vi "Tool-BLED112 GUI IntervalTime Cal.vi"() -> ()   [LabVIEW 2015]
uses:
  <vilib>/Analysis/baseanly.llb/Mean (DBL).vi
  <vilib>/Analysis/NI_AALBase.lvlib
panel:
  out "전체 시간(s)":dbl=17.30500000000029 format="%0.2f"
  out "평균 Interval time(ms)":dbl=49.87031700288185 format="%0.2f"
  out "Packet Length":i32=349
  out "Interval time":dbl(graph)=3.0
  in  "Log data &bled gui":string="2016.08.18 17:13:00.655 ble_evt_attclient_attribute_value connection: 0 (0x00) atthandle: 11 (0x000b) type: 1 (0x01) value:1fe8952003fc1fd90f20421d205d8a201abb0100\n2016.08.18 17:13:00.657 RX: 80190405000b0001141fe8952003fc1fd90f20421d205d8a201abb0100\n\n2016.08.18 17:13:00.658 ble_evt_attclient_attribute_value connection: 0 (0x00) atthandle: 15 (0x000f) type: 1 (0x01) value:02bcfe33fe4b0158ff4241a70000000000000000\n2016.08.18 17:13:00.659 RX: 80190405000f00011402bcfe33fe4b0158ff4241a70000000000000000\n\n2016.08.18 17:13:00.753 ble_evt_attclient_attribute_value connection: 0 (0x00) atthandle: 11 (0x000b) type: 1 (0x01) value:1fe8952003fa1fd910204218205d87201abe0100\n2016.08.18 17:13:00.754 RX: 80190405000b0001141fe8952003fa1fd910204218205d87201abe0100\n\n2016.08.18 17:13:00.758 ble_evt_attclient_attribute_value connection: 0 (0x00) atthandle: 15 (0x000f) type: 1 (0x01) value:02c4fe29fe48013bff5b41ac0000000000000000\n2016.08.18 17:13:00.759 RX: 80190405000f00011402c4fe29fe48013bff5b41ac0000000000000000\n\n2016.08.18 17:13:00.858 ble_evt_attclient_attribute_value connection: 0 (0x00) atthandle: 11 (0x000b) type: 1 (0x01) value:1fe8932003f91fd90e204217205d83201abc0100\n2016.08.18 17:13:00.859 RX: 80190405000b0001141fe8932003f91fd90e204217205d83201abc0100\n\n2016.08.18 17:13:00.860 ble_evt_attclient_attribute_value connection: 0 (0x00) atthandle: 15 (0x000f) type: 1 (0x01) value:02c8fe2efe470135ff6341b80000000000000000\n2016.08.18 17:13:00.862 RX: 80190405000f00011402c8fe2efe470135ff6341b80000000000000000\n\n2016.08.18 17:13:00.955 ble_evt_attclient_attribute_value connection: 0 (0x00) atthandle: 11 (0x000b) type: 1 (0x01) value:1fe8922003f51fd915204218205d87201aba0100\n2016.08.18 17:13:00.957 RX: 80190405000b0001141fe8922003f51fd915204218205d87201aba0100\n\n2016.08.18 17:13:00.958 ble_evt_attclient_attribute_value connection: 0 (0x00) atthandle: 15 (0x000f) type: 1 (0x01) value:02c8fe27fe4b013dff4741b70000000000000000\n2016.08.18 17:13:00.959 RX: 80190405000f00011402c8fe27fe4b013dff4741b70000000000000000\n\n2016.08.18 17:13:01.053 ble_evt_attclient_attribute_value connection: 0 (0x00) atthandle: 11 (0x000b) type: 1 (0x01) value:1fe8a02003f91fd91820421a205d8b201ab70100\n2016.08.18 17:13:01.055 RX: 80190405000b0001141fe8a02003f91fd91820421a205d8b201ab70100\n\n2016.08.18 17:13:01.060 ble_evt_attclient_attribute_value connection: 0 (0x00) atthandle: 15 (0x000f) type: 1 (0x01) value:02bbfe24fe4c0149ff2641b80000000000000000\n2016.08.18 17:13:01.061 RX: 80190405000f00011402bbfe24fe4c0149ff2641b80000000000000000\n\n2016.08.18 17:13:01.158 ble_evt_attclient_attribute_value connection: 0 (0x00) atthandle: 11 (0x000b) type: 1 (0x01) value:1fe8a02003fb1fd917204216205d86201ab40100\n2016.08.18 17:13:01.159 RX: 80190405000b0001141fe8a02003fb1fd917204216205d86201ab40100\n\n2016.08.18 17:13:01.160 ble_evt_attclient_attribute_value connection: 0 (0x00) atthandle: 15 (0x000f) type: 1 (0x01) value:02c1fe27fe4b014cff4541a90000000000000000\n2016.08.18 17:13:01.162 RX: 80190405000f00011402c1fe27fe4b014cff4541a90000000000000000\n\n2016.08.18 17:13:01.255 ble_evt_attclient_attribute_value connection: 0 (0x00) atthandle: 11 (0x000b) type: 1 (0x01) value:1fe8a02003f81fd91520421e205d85201ab30100\n2016.08.18 17:13:01.257 RX: 80190405000b0001141fe8a02003f81fd91520421e205d85201ab30100\n\n2016.08.18 17:13:01.258 ble_evt_attclient_attribute_value connection: 0 (0x00) atthandle: 15 (0x000f) type: 1 (0x01) value:02cafe24fe460141ff2f41c60000000000000000\n2016.08.18 17:13:01.259 RX: 80190405000f00011402cafe24fe460141ff2f41c60000000000000000\n\n2016.08.18 17:13:01.353 ble_evt_attclient_attribute_value connection: 0 (0x00) atthandle: 11 (0x000b) type: 1 (0x01) value:1fe89f2003f91fd916204221205d82201ab20100\n2016.08.18 17:13:01.355 RX: 80190405000b0001141fe89f2003f91fd916204221205d82201ab20100\n\n2016.08.18 17:13:01.356 ble_evt_attclient_attribute_value connection: 0 (0x00) atthandle: 15 (0x000f) type: 1 (0x01) value:02cafe2bfe4d0158ff4a41c30000000000000000\n2016.08.18 17:13:01.357 RX: 80190405000f00011402cafe2bfe4d0158ff4a41c30000000000000000\n\n2016.08.18 17:13:01.458 ble_evt_attclient_attribute_value connection: 0 (0x00) atthandle: 11 (0x000b) type: 1 (0x01) value:1fe8962003f41fd91420421c205d80201aab0100\n2016.08.18 17:13:01.459 RX: 80190405000b0001141fe8962003f41fd91420421c205d80201aab0100\n\n2016.08.18 17:13:01.460 ble_evt_attclient_attribute_value connection: 0 (0x00) atthandle: 15 (0x000f) type: 1 (0x01) value:02cafe28fe50011bff4941ab0000000000000000\n2016.08.18 17:13:01.462 RX: 80190405000f00011402cafe28fe50011bff4941ab0000000000000000\n\n2016.08.18 17:13:01.563 ble_evt_attclient_attribute_value connection: 0 (0x00) atthandle: 11 (0x000b) type: 1 (0x01) value:1fe8982003f91fd914204222205d88201aae0100\n2016.08.18 17:13:01.564 RX: 80190405000b0001141fe8982003f91fd914204222205d88201aae0100\n\n2016.08.18 17:13:01.565 ble_evt_attclient_attribute_value connection: 0 (0x00) atthandle: 15 (0x000f) type: 1 (0x01) value:02b6fe2ffe52014cff4541970000000000000000\n2016.08.18 17:13:01.567 RX: 80190405000f00011402b6fe2ffe52014cff4541970000000000000000\n\n2016.08.18 17:13:01.652 ble_evt_attclient_attribute_value connection: 0 (0x00) atthandle: 11 (0x000b) type: 1 (0x01) value:1fe89a2004001fd912204222205d8f201ab70100\n2016.08.18 17:13:01.654 RX: 80190405000b0001141fe89a2004001fd912204222205d8f201ab70100\n\n2016.08.18 17:13:01.660 ble_evt_attclient_attribute_value connection: 0 (0x00) atthandle: 15 (0x000f) type: 1 (0x01) value:02b8fe2cfe4d0158ff3c41aa0000000000000000\n2016.08.18 17:13:01.661 RX: 80190405000f00011402b8fe2cfe4d0158ff3c41aa0000000000000000\n\n2016.08.18 17:13:01.765 ble_evt_attclient_attribute_value connection: 0 (0x00) atthandle: 11 (0x000b) type: 1 (0x01) value:1fe8962003f91fd913204222205d8d201ab50100\n2016.08.18 17:13:01.767 RX: 80190405000b0001141fe8962003f91fd913204222205d8d201ab50100\n\n2016.08.18 17:13:01.768 ble_evt_attclient_attribute_value connection: 0 (0x00) atthandle: 15 (0x000f) type: 1 (0x01) value:02c9fe24fe450173ff2e41b40000000000000000\n2016.08.18 17:13:01.769 RX: 80190405000f00011402c9fe24fe450173ff2e41b40000000000000000\n\n2016.08.18 17:13:01.856 ble_evt_attclient_attribute_value connection: 0 (0x00) atthandle: 11 (0x000b) type: 1 (0x01) value:1fe89a2003f91fd911204220205d91201ab70100\n2016.08.18 17:13:01.858 RX: 80190405000b0001141fe89a2003f91fd911204220205d91201ab70100\n\n2016.08.18 17:13:01.862 ble_evt_attclient_attribute_value connection: 0 (0x00) atthandle: 15 (0x000f) type: 1 (0x01) value:02c2fe2afe460169ff4441d50000000000000000\n2016.08.18 17:13:01.863 RX: 80190405000f00011402c2fe2afe460169ff4441d50000000000000000\n\n2016.08.18 17:13:01.953 ble_evt_attclient_attribute_value connection: 0 (0x00) atthandle: 11 (0x000b) type: 1 (0x01) value:1fe8932003fa1fd90d20421b205d88201aab0100\n2016.08.18 17:13:01.954 RX: 80190405000b0001141fe8932003fa1fd90d20421b205d88201aab0100\n\n2016.08.18 17:13:01.955 ble_evt_attclient_attribute_value connection: 0 (0x00) atthandle: 15 (0x000f) type: 1 (0x01) value:02c9fe2cfe450161ff5f41c70000000000000000\n2016.08.18 17:13:01.957 RX: 80190405000f00011402c9fe2cfe450161ff5f41c70000000000000000\n\n2016.08.18 17:13:02.058 ble_evt_attclient_attribute_value connection: 0 (0x00) atthandle: 11 (0x000b) type: 1 (0x01) value:1fe8952003fa1fd91020421a205d8a201ab50100\n2016.08.18 17:13:02.059 RX: 80190405000b0001141fe8952003fa1fd91020421a205d8a201ab50100\n\n2016.08.18 17:13:02.060 ble_evt_attclient_attribute_value connection: 0 (0x00) atthandle: 15 (0x000f) type: 1 (0x01) value:02cbfe26fe41013cff3c41aa0000000000000000\n2016.08.18 17:13:02.062 RX: 80190405000f00011402cbfe26fe41013cff3c41aa0000000000000000\n\n2016.08.18 17:13:02.155 ble_evt_attclient_attribute_value connection: 0 (0x00) atthandle: 11 (0x000b) type: 1 (0x01) value:1fe8972003fb1fd913204217205d8e201ab40100\n2016.08.18 17:13:02.157 RX: 80190405000b0001141fe8972003fb1fd913204217205d8e201ab40100\n\n2016.08.18 17:13:02.158 ble_evt_attclient_attribute_value connection: 0 (0x00) atthandle: 15 (0x000f) type: 1 (0x01) value:02c7fe28fe41012dff3b41930000000000000000\n2016.08.18 17:13:02.159 RX: 80190405000f00011402c7fe28fe41012dff3b41930000000000000000\n\n2016.08.18 17:13:02.253 ble_evt_attclient_attribute_value connection: 0 (0x00) atthandle: 11 (0x000b) type: 1 (0x01) value:1fe8922003f31fd91620421c205d90201ab10100\n2016.08.18 17:13:02.254 RX: 80190405000b0001141fe8922003f31fd91620421c205d90201ab10100\n\n2016.08.18 17:13:02.256 ble_evt_attclient_attribute_value connection: 0 (0x00) atthandle: 15 (0x000f) type: 1 (0x01) value:02c5fe24fe44015aff3141820000000000000000\n2016.08.18 17:13:02.257 RX: 80190405000f00011402c5fe24fe44015aff3141820000000000000000\n\n2016.08.18 17:13:02.358 ble_evt_attclient_attribute_value connection: 0 (0x00) atthandle: 11 (0x000b) type: 1 (0x01) value:1fe8912003f21fd915204218205d8f201aaf0100\n2016.08.18 17:13:02.359 RX: 80190405000b0001141fe8912003f21fd915204218205d8f201aaf0100\n\n2016.08.18 17:13:02.360 ble_evt_attclient_attribute_value connection: 0 (0x00) atthandle: 15 (0x000f) type: 1 (0x01) value:02cbfe2dfe500170ff3c41a10000000000000000\n2016.08.18 17:13:02.362 RX: 80190405000f00011402cbfe2dfe500170ff3c41a10000000000000000\n\n2016.08.18 17:13:02.455 ble_evt_attclient_attribute_value connection: 0 (0x00) atthandle: 11 (0x000b) type: 1 (0x01) value:1fe88f2003f51fd916204218205d90201ab20100\n2016.08.18 17:13:02.457 RX: 80190405000b0001141fe88f2003f51fd916204218205d90201ab20100\n\n2016.08.18 17:13:02.458 ble_evt_attclient_attribute_value connection: 0 (0x00) atthandle: 15 (0x000f) type: 1 (0x01) value:02bdfe30fe500157ff5541b20000000000000000\n2016.08.18 17:13:02.459 RX: 80190405000f00011402bdfe30fe500157ff5541b20000000000000000\n\n2016.08.18 17:13:02.553 ble_evt_attclient_attribute_value connection: 0 (0x00) atthandle: 11 (0x000b) type: 1 (0x01) value:1fe88e2003ed1fd910204218205d92201ab30100\n2016.08.18 17:13:02.554 RX: 80190405000b0001141fe88e2003ed1fd910204218205d92201ab30100\n\n2016.08.18 17:13:02.555 ble_evt_attclient_attribute_value connection: 0 (0x00) atthandle: 15 (0x000f) type: 1 (0x01) value:02bcfe22fe510132ff5541930000000000000000\n2016.08.18 17:13:02.557 RX: 80190405000f00011402bcfe22fe510132ff5541930000000000000000\n\n2016.08.18 17:13:02.657 ble_evt_attclient_attribute_value connection: 0 (0x00) atthandle: 11 (0x000b) type: 1 (0x01) value:1fe88c2003ec1fd912204213205d8f201ab30100\n2016.08.18 17:13:02.659 RX: 80190405000b0001141fe88c2003ec1fd912204213205d8f201ab30100\n\n2016.08.18 17:13:02.672 ble_evt_attclient_attribute_value connection: 0 (0x00) atthandle: 15 (0x000f) type: 1 (0x01) value:02c6fe20fe500126ff2541c60000000000000000\n2016.08.18 17:13:02.673 RX: 80190405000f00011402c6fe20fe500126ff2541c60000000000000000\n\n2016.08.18 17:13:02.755 ble_evt_attclient_attribute_value connection: 0 (0x00) atthandle: 11 (0x000b) type: 1 (0x01) value:1fe8902003f11fd916204215205d91201ab40100\n2016.08.18 17:13:02.757 RX: 80190405000b0001141fe8902003f11fd916204215205d91201ab40100\n\n2016.08.18 17:13:02.758 ble_evt_attclient_attribute_value connection: 0 (0x00) atthandle: 15 (0x000f) type: 1 (0x01) value:02ccfe28fe470158ff3841a30000000000000000\n2016.08.18 17:13:02.759 RX: 80190405000f00011402ccfe28fe470158ff3841a30000000000000000\n\n2016.08.18 17:13:02.853 ble_evt_attclient_attribute_value connection: 0 (0x00) atthandle: 11 (0x000b) type: 1 (0x01) value:1fe88d2003f31fd915204218205d92201ab30100\n2016.08.18 17:13:02.854 RX: 80190405000b0001141fe88d2003f31fd915204218205d92201ab30100\n\n2016.08.18 17:13:02.855 ble_evt_attclient_attribute_value connection: 0 (0x00) atthandle: 15 (0x000f) type: 1 (0x01) value:02c7fe29fe520159ff3041a30000000000000000\n2016.08.18 17:13:02.857 RX: 80190405000f00011402c7fe29fe520159ff3041a30000000000000000\n\n2016.08.18 17:13:02.973 ble_evt_attclient_attribute_value connection: 0 (0x00) atthandle: 11 (0x000b) type: 1 (0x01) value:1fe88a2003ef1fd910204213205d94201ab30100\n2016.08.18 17:13:02.974 RX: 80190405000b0001141fe88a2003ef1fd910204213205d94201ab30100\n\n2016.08.18 17:13:02.975 ble_evt_attclient_attribute_value connection: 0 (0x00) atthandle: 15 (0x000f) type: 1 (0x01) value:02d3fe2efe490173ff4d419d0000000000000000\n2016.08.18 17:13:02.977 RX: 80190405000f00011402d3fe2efe490173ff4d419d0000000000000000\n\n2016.08.18 17:13:03.055 ble_evt_attclient_attribute_value connection: 0 (0x00) atthandle: 11 (0x000b) type: 1 (0x01) value:1fe88d2003f61fd91a204215205d9a201abb0100\n2016.08.18 17:13:03.057 RX: 80190405000b0001141fe88d2003f61fd91a204215205d9a201abb0100\n\n2016.08.18 17:13:03.058 ble_evt_attclient_attribute_value connection: 0 (0x00) atthandle: 15 (0x000f) type: 1 (0x01) value:02bbfe2ffe4c013cff5241c40000000000000000\n2016.08.18 17:13:03.059 RX: 80190405000f00011402bbfe2ffe4c013cff5241c40000000000000000\n\n2016.08.18 17:13:03.153 ble_evt_attclient_attribute_value connection: 0 (0x00) atthandle: 11 (0x000b) type: 1 (0x01) value:1fe8942003fd1fd91d204216205d9e201ac20100\n2016.08.18 17:13:03.154 RX: 80190405000b0001141fe8942003fd1fd91d204216205d9e201ac20100\n\n2016.08.18 17:13:03.156 ble_evt_attclient_attribute_value connection: 0 (0x00) atthandle: 15 (0x000f) type: 1 (0x01) value:02c0fe27fe4e0133ff4c41bc0000000000000000\n2016.08.18 17:13:03.157 RX: 80190405000f00011402c0fe27fe4e0133ff4c41bc0000000000000000\n\n2016.08.18 17:13:03.258 ble_evt_attclient_attribute_value connection: 0 (0x00) atthandle: 11 (0x000b) type: 1 (0x01) value:1fe8962004041fd92220421c205d9e201ac40100\n2016.08.18 17:13:03.260 RX: 80190405000b0001141fe8962004041fd92220421c205d9e201ac40100\n\n2016.08.18 17:13:03.264 ble_evt_attclient_attribute_value connection: 0 (0x00) atthandle: 15 (0x000f) type: 1 (0x01) value:02c4fe21fe430149ff3741b40000000000000000\n2016.08.18 17:13:03.266 RX: 80190405000f00011402c4fe21fe430149ff3741b40000000000000000\n\n2016.08.18 17:13:03.355 ble_evt_attclient_attribute_value connection: 0 (0x00) atthandle: 11 (0x000b) type: 1 (0x01) value:1fe8942004021fd91d204218205d9d201abc0100\n2016.08.18 17:13:03.357 RX: 80190405000b0001141fe8942004021fd91d204218205d9d201abc0100\n\n2016.08.18 17:13:03.358 ble_evt_attclient_attribute_value connection: 0 (0x00) atthandle: 15 (0x000f) type: 1 (0x01) value:02b6fe2bfe410142ff3d41a30000000000000000\n2016.08.18 17:13:03.359 RX: 80190405000f00011402b6fe2bfe410142ff3d41a30000000000000000\n\n2016.08.18 17:13:03.453 ble_evt_attclient_attribute_value connection: 0 (0x00) atthandle: 11 (0x000b) type: 1 (0x01) value:1fe89a2004041fd92320421d205da1201ac00100\n2016.08.18 17:13:03.455 RX: 80190405000b0001141fe89a2004041fd92320421d205da1201ac00100\n\n2016.08.18 17:13:03.456 ble_evt_attclient_attribute_value connection: 0 (0x00) atthandle: 15 (0x000f) type: 1 (0x01) value:02b7fe33fe470160ff2d41b60000000000000000\n2016.08.18 17:13:03.457 RX: 80190405000f00011402b7fe33fe470160ff2d41b60000000000000000\n\n2016.08.18 17:13:03.558 ble_evt_attclient_attribute_value connection: 0 (0x00) atthandle: 11 (0x000b) type: 1 (0x01) value:1fe8942003f91fd91c204217205d93201ab40100\n2016.08.18 17:13:03.559 RX: 80190405000b0001141fe8942003f91fd91c204217205d93201ab40100\n\n2016.08.18 17:13:03.560 ble_evt_attclient_attribute_value connection: 0 (0x00) atthandle: 15 (0x000f) type: 1 (0x01) value:02bdfe2bfe49013cff5c41c10000000000000000\n2016.08.18 17:13:03.562 RX: 80190405000f00011402bdfe2bfe49013cff5c41c10000000000000000\n\n2016.08.18 17:13:03.655 ble_evt_attclient_attribute_value connection: 0 (0x00) atthandle: 11 (0x000b) type: 1 (0x01) value:1fe8982003fe1fd91f20421a205d97201ab90100\n2016.08.18 17:13:03.657 RX: 80190405000b0001141fe8982003fe1fd91f20421a205d97201ab90100\n\n2016.08.18 17:13:03.658 ble_evt_attclient_attribute_value connection: 0 (0x00) atthandle: 15 (0x000f) type: 1 (0x01) value:02ccfe25fe4a0124ff5341b50000000000000000\n2016.08.18 17:13:03.659 RX: 80190405000f00011402ccfe25fe4a0124ff5341b50000000000000000\n\n2016.08.18 17:13:03.753 ble_evt_attclient_attribute_value connection: 0 (0x00) atthandle: 11 (0x000b) type: 1 (0x01) value:1fe8942003fb1fd919204215205d92201ab10100\n2016.08.18 17:13:03.754 RX: 80190405000b0001141fe8942003fb1fd919204215205d92201ab10100\n\n2016.08.18 17:13:03.756 ble_evt_attclient_attribute_value connection: 0 (0x00) atthandle: 15 (0x000f) type: 1 (0x01) value:02befe2afe40012bff4741c00000000000000000\n2016.08.18 17:13:03.757 RX: 80190405000f00011402befe2afe40012bff4741c00000000000000000\n\n2016.08.18 17:13:03.858 ble_evt_attclient_attribute_value connection: 0 (0x00) atthandle: 11 (0x000b) type: 1 (0x01) value:1fe8962003fa1fd916204212205d8c201aba0100\n2016.08.18 17:13:03.859 RX: 80190405000b0001141fe8962003fa1fd916204212205d8c201aba0100\n\n2016.08.18 17:13:03.860 ble_evt_attclient_attribute_value connection: 0 (0x00) atthandle: 15 (0x000f) type: 1 (0x01) value:02b2fe2efe4a0148ff3341aa0000000000000000\n2016.08.18 17:13:03.861 RX: 80190405000f00011402b2fe2efe4a0148ff3341aa0000000000000000\n\n2016.08.18 17:13:03.955 ble_evt_attclient_attribute_value connection: 0 (0x00) atthandle: 11 (0x000b) type: 1 (0x01) value:1fe8912003f31fd912204212205d8a201ab90100\n2016.08.18 17:13:03.957 RX: 80190405000b0001141fe8912003f31fd912204212205d8a201ab90100\n\n2016.08.18 17:13:03.958 ble_evt_attclient_attribute_value connection: 0 (0x00) atthandle: 15 (0x000f) type: 1 (0x01) value:02c5fe2afe4e0174ff2541a90000000000000000\n2016.08.18 17:13:03.959 RX: 80190405000f00011402c5fe2afe4e0174ff2541a90000000000000000\n\n2016.08.18 17:13:04.053 ble_evt_attclient_attribute_value connection: 0 (0x00) atthandle: 11 (0x000b) type: 1 (0x01) value:1fe8972003f71fd91a20421b205d90201ac10100\n2016.08.18 17:13:04.054 RX: 80190405000b0001141fe8972003f71fd91a20421b205d90201ac10100\n\n2016.08.18 17:13:04.056 ble_evt_attclient_attribute_value connection: 0 (0x00) atthandle: 15 (0x000f) type: 1 (0x01) value:02c8fe25fe47015aff4b41cb0000000000000000\n2016.08.18 17:13:04.057 RX: 80190405000f00011402c8fe25fe47015aff4b41cb0000000000000000\n\n2016.08.18 17:13:04.158 ble_evt_attclient_attribute_value connection: 0 (0x00) atthandle: 11 (0x000b) type: 1 (0x01) value:1fe89c2003f81fd91c20421c205d93201ac20100\n2016.08.18 17:13:04.159 RX: 80190405000b0001141fe89c2003f81fd91c20421c205d93201ac20100\n\n2016.08.18 17:13:04.160 ble_evt_attclient_attribute_value connection: 0 (0x00) atthandle: 15 (0x000f) type: 1 (0x01) value:02bcfe2afe420143ff6e41ca0000000000000000\n2016.08.18 17:13:04.161 RX: 80190405000f00011402bcfe2afe420143ff6e41ca0000000000000000\n\n2016.08.18 17:13:04.262 ble_evt_attclient_attribute_value connection: 0 (0x00) atthandle: 11 (0x000b) type: 1 (0x01) value:1fe89b2003f91fd91b204220205d93201ac10100\n2016.08.18 17:13:04.263 RX: 80190405000b0001141fe89b2003f91fd91b204220205d93201ac10100\n\n2016.08.18 17:13:04.265 ble_evt_attclient_attribute_value connection: 0 (0x00) atthandle: 15 (0x000f) type: 1 (0x01) value:02befe31fe520132ff4e41a30000000000000000\n2016.08.18 17:13:04.266 RX: 80190405000f00011402befe31fe520132ff4e41a30000000000000000\n\n2016.08.18 17:13:04.353 ble_evt_attclient_attribute_value connection: 0 (0x00) atthandle: 11 (0x000b) type: 1 (0x01) value:1fe8942003f51fd916204217205d8f201abd0100\n2016.08.18 17:13:04.354 RX: 80190405000b0001141fe8942003f51fd916204217205d8f201abd0100\n\n2016.08.18 17:13:04.355 ble_evt_attclient_attribute_value connection: 0 (0x00) atthandle: 15 (0x000f) type: 1 (0x01) value:02c9fe26fe450146ff1941b10000000000000000\n2016.08.18 17:13:04.357 RX: 80190405000f00011402c9fe26fe450146ff1941b10000000000000000\n\n2016.08.18 17:13:04.458 ble_evt_attclient_attribute_value connection: 0 (0x00) atthandle: 11 (0x000b) type: 1 (0x01) value:1fe8952003f91fd917204216205d8d201ac00100\n2016.08.18 17:13:04.459 RX: 80190405000b0001141fe8952003f91fd917204216205d8d201ac00100\n\n2016.08.18 17:13:04.460 ble_evt_attclient_attribute_value connection: 0 (0x00) atthandle: 15 (0x000f) type: 1 (0x01) value:02bcfe29fe550157ff3741c10000000000000000\n2016.08.18 17:13:04.461 RX: 80190405000f00011402bcfe29fe550157ff3741c10000000000000000\n\n2016.08.18 17:13:04.563 ble_evt_attclient_attribute_value connection: 0 (0x00) atthandle: 11 (0x000b) type: 1 (0x01) value:1fe8942003f11fd919204213205d8a201abd0100\n2016.08.18 17:13:04.565 RX: 80190405000b0001141fe8942003f11fd919204213205d8a201abd0100\n\n2016.08.18 17:13:04.566 ble_evt_attclient_attribute_value connection: 0 (0x00) atthandle: 15 (0x000f) type: 1 (0x01) value:02c0fe31fe440171ff4a41b60000000000000000\n2016.08.18 17:13:04.567 RX: 80190405000f00011402c0fe31fe440171ff4a41b60000000000000000\n\n2016.08.18 17:13:04.660 ble_evt_attclient_attribute_value connection: 0 (0x00) atthandle: 11 (0x000b) type: 1 (0x01) value:1fe8942003ef1fd91e204216205d8d201abd0100\n2016.08.18 17:13:04.661 RX: 80190405000b0001141fe8942003ef1fd91e204216205d8d201abd0100\n\n2016.08.18 17:13:04.667 ble_evt_attclient_attribute_value connection: 0 (0x00) atthandle: 15 (0x000f) type: 1 (0x01) value:02bbfe2dfe420147ff4f41ba0000000000000000\n2016.08.18 17:13:04.668 RX: 80190405000f00011402bbfe2dfe420147ff4f41ba0000000000000000\n\n2016.08.18 17:13:04.765 ble_evt_attclient_attribute_value connection: 0 (0x00) atthandle: 11 (0x000b) type: 1 (0x01) value:1fe89e2003f31fd922204218205d90201abe0100\n2016.08.18 17:13:04.767 RX: 80190405000b0001141fe89e2003f31fd922204218205d90201abe0100\n\n2016.08.18 17:13:04.768 ble_evt_attclient_attribute_value connection: 0 (0x00) atthandle: 15 (0x000f) type: 1 (0x01) value:02c3fe35fe460144ff6641b60000000000000000\n2016.08.18 17:13:04.769 RX: 80190405000f00011402c3fe35fe460144ff6641b60000000000000000\n\n2016.08.18 17:13:04.855 ble_evt_attclient_attribute_value connection: 0 (0x00) atthandle: 11 (0x000b) type: 1 (0x01) value:1fe89d2003f11fd91b204217205d8d201ab80100\n2016.08.18 17:13:04.857 RX: 80190405000b0001141fe89d2003f11fd91b204217205d8d201ab80100\n\n2016.08.18 17:13:04.858 ble_evt_attclient_attribute_value connection: 0 (0x00) atthandle: 15 (0x000f) type: 1 (0x01) value:02b9fe2dfe460140ff5541aa0000000000000000\n2016.08.18 17:13:04.859 RX: 80190405000f00011402b9fe2dfe460140ff5541aa0000000000000000\n\n2016.08.18 17:13:04.967 ble_evt_attclient_attribute_value connection: 0 (0x00) atthandle: 11 (0x000b) type: 1 (0x01) value:1fe89f2003ed1fd91a204218205d8b201ab20100\n2016.08.18 17:13:04.969 RX: 80190405000b0001141fe89f2003ed1fd91a204218205d8b201ab20100\n\n2016.08.18 17:13:04.970 ble_evt_attclient_attribute_value connection: 0 (0x00) atthandle: 15 (0x000f) type: 1 (0x01) value:02bdfe30fe49015dff3141b40000000000000000\n2016.08.18 17:13:04.971 RX: 80190405000f00011402bdfe30fe49015dff3141b40000000000000000\n\n2016.08.18 17:13:05.065 ble_evt_attclient_attribute_value connection: 0 (0x00) atthandle: 11 (0x000b) type: 1 (0x01) value:1fe89d2003ed1fd915204217205d85201aaf0100\n2016.08.18 17:13:05.067 RX: 80190405000b0001141fe89d2003ed1fd915204217205d85201aaf0100\n\n2016.08.18 17:13:05.068 ble_evt_attclient_attribute_value connection: 0 (0x00) atthandle: 15 (0x000f) type: 1 (0x01) value:02c3fe33fe530159ff3041c30000000000000000\n2016.08.18 17:13:05.069 RX: 80190405000f00011402c3fe33fe530159ff3041c30000000000000000\n\n2016.08.18 17:13:05.155 ble_evt_attclient_attribute_value connection: 0 (0x00) atthandle: 11 (0x000b) type: 1 (0x01) value:1fe89c2003f01fd91720421a205d87201ab00100\n2016.08.18 17:13:05.156 RX: 80190405000b0001141fe89c2003f01fd91720421a205d87201ab00100\n\n2016.08.18 17:13:05.162 ble_evt_attclient_attribute_value connection: 0 (0x00) atthandle: 15 (0x000f) type: 1 (0x01) value:02c1fe2dfe4b0174ff3541a80000000000000000\n2016.08.18 17:13:05.163 RX: 80190405000f00011402c1fe2dfe4b0174ff3541a80000000000000000\n\n2016.08.18 17:13:05.267 ble_evt_attclient_attribute_value connection: 0 (0x00) atthandle: 11 (0x000b) type: 1 (0x01) value:1fe8992003f11fd91520421d205d8b201aae0100\n2016.08.18 17:13:05.269 RX: 80190405000b0001141fe8992003f11fd91520421d205d8b201aae0100\n\n2016.08.18 17:13:05.270 ble_evt_attclient_attribute_value connection: 0 (0x00) atthandle: 15 (0x000f) type: 1 (0x01) value:02b0fe34fe550153ff5841b20000000000000000\n2016.08.18 17:13:05.271 RX: 80190405000f00011402b0fe34fe550153ff5841b20000000000000000\n\n2016.08.18 17:13:05.367 ble_evt_attclient_attribute_value connection: 0 (0x00) atthandle: 11 (0x000b) type: 1 (0x01) value:1fe89d2003fb1fd917204228205d99201ac00100\n2016.08.18 17:13:05.368 RX: 80190405000b0001141fe89d2003fb1fd917204228205d99201ac00100\n\n2016.08.18 17:13:05.369 ble_evt_attclient_attribute_value connection: 0 (0x00) atthandle: 15 (0x000f) type: 1 (0x01) value:02affe26fe530136ff5d41bd0000000000000000\n2016.08.18 17:13:05.371 RX: 80190405000f00011402affe26fe530136ff5d41bd0000000000000000\n\n2016.08.18 17:13:05.455 ble_evt_attclient_attribute_value connection: 0 (0x00) atthandle: 11 (0x000b) type: 1 (0x01) value:1fe89b2003fa1fd919204223205d99201abe0100\n2016.08.18 17:13:05.457 RX: 80190405000b0001141fe89b2003fa1fd919204223205d99201abe0100\n\n2016.08.18 17:13:05.458 ble_evt_attclient_attribute_value connection: 0 (0x00) atthandle: 15 (0x000f) type: 1 (0x01) value:02ccfe2efe41012dff4541c50000000000000000\n2016.08.18 17:13:05.459 RX: 80190405000f00011402ccfe2efe41012dff4541c50000000000000000\n\n2016.08.18 17:13:05.552 ble_evt_attclient_attribute_value connection: 0 (0x00) atthandle: 11 (0x000b) type: 1 (0x01) value:1fe8982003f51fd913204222205d97201aba0100\n2016.08.18 17:13:05.553 RX: 80190405000b0001141fe8982003f51fd913204222205d97201aba0100\n\n2016.08.18 17:13:05.567 ble_evt_attclient_attribute_value connection: 0 (0x00) atthandle: 15 (0x000f) type: 1 (0x01) value:02befe25fe4c0159ff2141b30000000000000000\n2016.08.18 17:13:05.568 RX: 80190405000f00011402befe25fe4c0159ff2141b30000000000000000\n\n2016.08.18 17:13:05.672 ble_evt_attclient_attribute_value connection: 0 (0x00) atthandle: 11 (0x000b) type: 1 (0x01) value:1fe88f2003f21fd90e20421b205d8d201ab20100\n2016.08.18 17:13:05.674 RX: 80190405000b0001141fe88f2003f21fd90e20421b205d8d201ab20100\n\n2016.08.18 17:13:05.675 ble_evt_attclient_attribute_value connection: 0 (0x00) atthandle: 15 (0x000f) type: 1 (0x01) value:02c2fe28fe4a0156ff3041c50000000000000000\n2016.08.18 17:13:05.677 RX: 80190405000f00011402c2fe28fe4a0156ff3041c50000000000000000\n\n2016.08.18 17:13:05.755 ble_evt_attclient_attribute_value connection: 0 (0x00) atthandle: 11 (0x000b) type: 1 (0x01) value:1fe8912003f61fd91420421c205d94201ab60100\n2016.08.18 17:13:05.757 RX: 80190405000b0001141fe8912003f61fd91420421c205d94201ab60100\n\n2016.08.18 17:13:05.758 ble_evt_attclient_attribute_value connection: 0 (0x00) atthandle: 15 (0x000f) type: 1 (0x01) value:02c4fe29fe40015eff4041c20000000000000000\n2016.08.18 17:13:05.759 RX: 80190405000f00011402c4fe29fe40015eff4041c20000000000000000\n\n2016.08.18 17:13:05.852 ble_evt_attclient_attribute_value connection: 0 (0x00) atthandle: 11 (0x000b) type: 1 (0x01) value:1fe8932003f71fd91a20421a205d98201ab60100\n2016.08.18 17:13:05.853 RX: 80190405000b0001141fe8932003f71fd91a20421a205d98201ab60100\n\n2016.08.18 17:13:05.874 ble_evt_attclient_attribute_value connection: 0 (0x00) atthandle: 15 (0x000f) type: 1 (0x01) value:02c9fe25fe4d0146ff5841b70000000000000000\n2016.08.18 17:13:05.876 RX: 80190405000f00011402c9fe25fe4d0146ff5841b70000000000000000\n\n2016.08.18 17:13:05.957 ble_evt_attclient_attribute_value connection: 0 (0x00) atthandle: 11 (0x000b) type: 1 (0x01) value:1fe8902003f41fd919204223205d98201ab80100\n2016.08.18 17:13:05.959 RX: 80190405000b0001141fe8902003f41fd919204223205d98201ab80100\n\n2016.08.18 17:13:05.960 ble_evt_attclient_attribute_value connection: 0 (0x00) atthandle: 15 (0x000f) type: 1 (0x01) value:02cafe2dfe58012bff4641af0000000000000000\n2016.08.18 17:13:05.961 RX: 80190405000f00011402cafe2dfe58012bff4641af0000000000000000\n\n2016.08.18 17:13:06.056 ble_evt_attclient_attribute_value connection: 0 (0x00) atthandle: 11 (0x000b) type: 1 (0x01) value:1fe8912003f51fd91a204220205d98201ab70100\n2016.08.18 17:13:06.058 RX: 80190405000b0001141fe8912003f51fd91a204220205d98201ab70100\n\n2016.08.18 17:13:06.059 ble_evt_attclient_attribute_value connection: 0 (0x00) atthandle: 15 (0x000f) type: 1 (0x01) value:02befe25fe4b012bff2f41c80000000000000000\n2016.08.18 17:13:06.060 RX: 80190405000f00011402befe25fe4b012bff2f41c80000000000000000\n\n2016.08.18 17:13:06.153 ble_evt_attclient_attribute_value connection: 0 (0x00) atthandle: 11 (0x000b) type: 1 (0x01) value:1fe8912003f61fd91b20421f205d99201ab40100\n2016.08.18 17:13:06.154 RX: 80190405000b0001141fe8912003f61fd91b20421f205d99201ab40100\n\n2016.08.18 17:13:06.160 ble_evt_attclient_attribute_value connection: 0 (0x00) atthandle: 15 (0x000f) type: 1 (0x01) value:02bcfe28fe53015eff1341ae0000000000000000\n2016.08.18 17:13:06.162 RX: 80190405000f00011402bcfe28fe53015eff1341ae0000000000000000\n\n2016.08.18 17:13:06.258 ble_evt_attclient_attribute_value connection: 0 (0x00) atthandle: 11 (0x000b) type: 1 (0x01) value:1fe88d2003f01fd91520421c205d95201ab00100\n2016.08.18 17:13:06.260 RX: 80190405000b0001141fe88d2003f01fd91520421c205d95201ab00100\n\n2016.08.18 17:13:06.261 ble_evt_attclient_attribute_value connection: 0 (0x00) atthandle: 15 (0x000f) type: 1 (0x01) value:02b6fe2dfe490165ff3c41b30000000000000000\n2016.08.18 17:13:06.263 RX: 80190405000f00011402b6fe2dfe490165ff3c41b30000000000000000\n\n2016.08.18 17:13:06.356 ble_evt_attclient_attribute_value connection: 0 (0x00) atthandle: 11 (0x000b) type: 1 (0x01) value:1fe88b2003eb1fd915204217205d90201aaf0100\n2016.08.18 17:13:06.358 RX: 80190405000b0001141fe88b2003eb1fd915204217205d90201aaf0100\n\n2016.08.18 17:13:06.359 ble_evt_attclient_attribute_value connection: 0 (0x00) atthandle: 15 (0x000f) type: 1 (0x01) value:02c4fe2afe4c013eff6441e60000000000000000\n2016.08.18 17:13:06.360 RX: 80190405000f00011402c4fe2afe4c013eff6441e60000000000000000\n\n2016.08.18 17:13:06.453 ble_evt_attclient_attribute_value connection: 0 (0x00) atthandle: 11 (0x000b) type: 1 (0x01) value:1fe88a2003ec1fd914204218205d8f201aad0100\n2016.08.18 17:13:06.454 RX: 80190405000b0001141fe88a2003ec1fd914204218205d8f201aad0100\n\n2016.08.18 17:13:06.460 ble_evt_attclient_attribute_value connection: 0 (0x00) atthandle: 15 (0x000f) type: 1 (0x01) value:02b7fe2afe540145ff6441cf0000000000000000\n2016.08.18 17:13:06.462 RX: 80190405000f00011402b7fe2afe540145ff6441cf0000000000000000\n\n2016.08.18 17:13:06.558 ble_evt_attclient_attribute_value connection: 0 (0x00) atthandle: 11 (0x000b) type: 1 (0x01) value:1fe8862003ed1fd914204218205d92201aab0100\n2016.08.18 17:13:06.560 RX: 80190405000b0001141fe8862003ed1fd914204218205d92201aab0100\n\n2016.08.18 17:13:06.561 ble_evt_attclient_attribute_value connection: 0 (0x00) atthandle: 15 (0x000f) type: 1 (0x01) value:02c3fe22fe46011fff2941ae0000000000000000\n2016.08.18 17:13:06.562 RX: 80190405000f00011402c3fe22fe46011fff2941ae0000000000000000\n\n2016.08.18 17:13:06.656 ble_evt_attclient_attribute_value connection: 0 (0x00) atthandle: 11 (0x000b) type: 1 (0x01) value:1fe8892003f01fd910204219205d98201ab30100\n2016.08.18 17:13:06.658 RX: 80190405000b0001141fe8892003f01fd910204219205d98201ab30100\n\n2016.08.18 17:13:06.659 ble_evt_attclient_attribute_value connection: 0 (0x00) atthandle: 15 (0x000f) type: 1 (0x01) value:02bffe26fe520152ff2841910000000000000000\n2016.08.18 17:13:06.660 RX: 80190405000f00011402bffe26fe520152ff2841910000000000000000\n\n2016.08.18 17:13:06.761 ble_evt_attclient_attribute_value connection: 0 (0x00) atthandle: 11 (0x000b) type: 1 (0x01) value:1fe88b2003f31fd91720421b205d9b201ab60100\n2016.08.18 17:13:06.762 RX: 80190405000b0001141fe88b2003f31fd91720421b205d9b201ab60100\n\n2016.08.18 17:13:06.764 ble_evt_attclient_attribute_value connection: 0 (0x00) atthandle: 15 (0x000f) type: 1 (0x01) value:02bcfe2afe4f0155ff3641a90000000000000000\n2016.08.18 17:13:06.765 RX: 80190405000f00011402bcfe2afe4f0155ff3641a90000000000000000\n\n2016.08.18 17:13:06.858 ble_evt_attclient_attribute_value connection: 0 (0x00) atthandle: 11 (0x000b) type: 1 (0x01) value:1fe8952003fa1fd91a20421e205d9e201ac40100\n2016.08.18 17:13:06.860 RX: 80190405000b0001141fe8952003fa1fd91a20421e205d9e201ac40100\n\n2016.08.18 17:13:06.861 ble_evt_attclient_attribute_value connection: 0 (0x00) atthandle: 15 (0x000f) type: 1 (0x01) value:02b9fe3afe500146ff4241b60000000000000000\n2016.08.18 17:13:06.862 RX: 80190405000f00011402b9fe3afe500146ff4241b60000000000000000\n\n2016.08.18 17:13:06.956 ble_evt_attclient_attribute_value connection: 0 (0x00) atthandle: 11 (0x000b) type: 1 (0x01) value:1fe8952004001fd91920421d205d9e201ac20100\n2016.08.18 17:13:06.957 RX: 80190405000b0001141fe8952004001fd91920421d205d9e201ac20100\n\n2016.08.18 17:13:06.958 ble_evt_attclient_attribute_value connection: 0 (0x00) atthandle: 15 (0x000f) type: 1 (0x01) value:02bffe30fe500153ff5f41a40000000000000000\n2016.08.18 17:13:06.960 RX: 80190405000f00011402bffe30fe500153ff5f41a40000000000000000\n\n2016.08.18 17:13:07.061 ble_evt_attclient_attribute_value connection: 0 (0x00) atthandle: 11 (0x000b) type: 1 (0x01) value:1fe8932003ff1fd91c20421c205da1201ac40100\n2016.08.18 17:13:07.062 RX: 80190405000b0001141fe8932003ff1fd91c20421c205da1201ac40100\n\n2016.08.18 17:13:07.063 ble_evt_attclient_attribute_value connection: 0 (0x00) atthandle: 15 (0x000f) type: 1 (0x01) value:02bdfe21fe4d0146ff4541c70000000000000000\n2016.08.18 17:13:07.065 RX: 80190405000f00011402bdfe21fe4d0146ff4541c70000000000000000\n\n2016.08.18 17:13:07.166 ble_evt_attclient_attribute_value connection: 0 (0x00) atthandle: 11 (0x000b) type: 1 (0x01) value:1fe8972003ff1fd91e204220205da1201abe0100\n2016.08.18 17:13:07.167 RX: 80190405000b0001141fe8972003ff1fd91e204220205da1201abe0100\n\n2016.08.18 17:13:07.168 ble_evt_attclient_attribute_value connection: 0 (0x00) atthandle: 15 (0x000f) type: 1 (0x01) value:02c5fe24fe4e0140ff21419d0000000000000000\n2016.08.18 17:13:07.170 RX: 80190405000f00011402c5fe24fe4e0140ff21419d0000000000000000\n\n2016.08.18 17:13:07.264 ble_evt_attclient_attribute_value connection: 0 (0x00) atthandle: 11 (0x000b) type: 1 (0x01) value:1fe8982003fe1fd91d204220205d9d201abf0100\n2016.08.18 17:13:07.265 RX: 80190405000b0001141fe8982003fe1fd91d204220205d9d201abf0100\n\n2016.08.18 17:13:07.266 ble_evt_attclient_attribute_value connection: 0 (0x00) atthandle: 15 (0x000f) type: 1 (0x01) value:02c4fe2ffe450152ff1d41a10000000000000000\n2016.08.18 17:13:07.268 RX: 80190405000f00011402c4fe2ffe450152ff1d41a10000000000000000\n\n2016.08.18 17:13:07.361 ble_evt_attclient_attribute_value connection: 0 (0x00) atthandle: 11 (0x000b) type: 1 (0x01) value:1fe89a2003fc1fd91c20421f205da0201abe0100\n2016.08.18 17:13:07.362 RX: 80190405000b0001141fe89a2003fc1fd91c20421f205da0201abe0100\n\n2016.08.18 17:13:07.364 ble_evt_attclient_attribute_value connection: 0 (0x00) atthandle: 15 (0x000f) type: 1 (0x01) value:02bffe21fe420156ff2f41a80000000000000000\n2016.08.18 17:13:07.365 RX: 80190405000f00011402bffe21fe420156ff2f41a80000000000000000\n\n2016.08.18 17:13:07.458 ble_evt_attclient_attribute_value connection: 0 (0x00) atthandle: 11 (0x000b) type: 1 (0x01) value:1fe89a2003fa1fd91520421c205d98201ab90100\n2016.08.18 17:13:07.460 RX: 80190405000b0001141fe89a2003fa1fd91520421c205d98201ab90100\n\n2016.08.18 17:13:07.461 ble_evt_attclient_attribute_value connection: 0 (0x00) atthandle: 15 (0x000f) type: 1 (0x01) value:02cbfe30fe42014dff6241b00000000000000000\n2016.08.18 17:13:07.462 RX: 80190405000f00011402cbfe30fe42014dff6241b00000000000000000\n\n2016.08.18 17:13:07.563 ble_evt_attclient_attribute_value connection: 0 (0x00) atthandle: 11 (0x000b) type: 1 (0x01) value:1fe8962003f71fd911204214205d8e201abe0100\n2016.08.18 17:13:07.565 RX: 80190405000b0001141fe8962003f71fd911204214205d8e201abe0100\n\n2016.08.18 17:13:07.566 ble_evt_attclient_attribute_value connection: 0 (0x00) atthandle: 15 (0x000f) type: 1 (0x01) value:02bafe26fe4f0137ff5b41cf0000000000000000\n2016.08.18 17:13:07.567 RX: 80190405000f00011402bafe26fe4f0137ff5b41cf0000000000000000\n\n2016.08.18 17:13:07.662 ble_evt_attclient_attribute_value connection: 0 (0x00) atthandle: 11 (0x000b) type: 1 (0x01) value:1fe8972003f41fd91320421b205d92201ac30100\n2016.08.18 17:13:07.663 RX: 80190405000b0001141fe8972003f41fd91320421b205d92201ac30100\n\n2016.08.18 17:13:07.669 ble_evt_attclient_attribute_value connection: 0 (0x00) atthandle: 15 (0x000f) type: 1 (0x01) value:02c5fe38fe540137ff2d41b20000000000000000\n2016.08.18 17:13:07.671 RX: 80190405000f00011402c5fe38fe540137ff2d41b20000000000000000\n\n2016.08.18 17:13:07.758 ble_evt_attclient_attribute_value connection: 0 (0x00) atthandle: 11 (0x000b) type: 1 (0x01) value:1fe8992003f61fd913204221205d93201ac60100\n2016.08.18 17:13:07.760 RX: 80190405000b0001141fe8992003f61fd913204221205d93201ac60100\n\n2016.08.18 17:13:07.761 ble_evt_attclient_attribute_value connection: 0 (0x00) atthandle: 15 (0x000f) type: 1 (0x01) value:02bbfe29fe580149ff2b41890000000000000000\n2016.08.18 17:13:07.762 RX: 80190405000f00011402bbfe29fe580149ff2b41890000000000000000\n\n2016.08.18 17:13:07.856 ble_evt_attclient_attribute_value connection: 0 (0x00) atthandle: 11 (0x000b) type: 1 (0x01) value:1fe89a2003f51fd915204221205d96201ac50100\n2016.08.18 17:13:07.857 RX: 80190405000b0001141fe89a2003f51fd915204221205d96201ac50100\n\n2016.08.18 17:13:07.858 ble_evt_attclient_attribute_value connection: 0 (0x00) atthandle: 15 (0x000f) type: 1 (0x01) value:02b0fe29fe4b0147ff3541a00000000000000000\n2016.08.18 17:13:07.860 RX: 80190405000f00011402b0fe29fe4b0147ff3541a00000000000000000\n\n2016.08.18 17:13:07.961 ble_evt_attclient_attribute_value connection: 0 (0x00) atthandle: 11 (0x000b) type: 1 (0x01) value:1fe89b2003f51fd917204226205d98201ac10100\n2016.08.18 17:13:07.962 RX: 80190405000b0001141fe89b2003f51fd917204226205d98201ac10100\n\n2016.08.18 17:13:07.963 ble_evt_attclient_attribute_value connection: 0 (0x00) atthandle: 15 (0x000f) type: 1 (0x01) value:02c3fe34fe47017bff3e419d0000000000000000\n2016.08.18 17:13:07.965 RX: 80190405000f00011402c3fe34fe47017bff3e419d0000000000000000\n\n2016.08.18 17:13:08.058 ble_evt_attclient_attribute_value connection: 0 (0x00) atthandle: 11 (0x000b) type: 1 (0x01) value:1fe8992003f71fd915204222205d94201abd0100\n2016.08.18 17:13:08.060 RX: 80190405000b0001141fe8992003f71fd915204222205d94201abd0100\n\n2016.08.18 17:13:08.061 ble_evt_attclient_attribute_value connection: 0 (0x00) atthandle: 15 (0x000f) type: 1 (0x01) value:02b0fe2bfe4b0158ff5041cf0000000000000000\n2016.08.18 17:13:08.062 RX: 80190405000f00011402b0fe2bfe4b0158ff5041cf0000000000000000\n\n2016.08.18 17:13:08.155 ble_evt_attclient_attribute_value connection: 0 (0x00) atthandle: 11 (0x000b) type: 1 (0x01) value:1fe8962003f51fd916204220205d8f201ac10100\n2016.08.18 17:13:08.157 RX: 80190405000b0001141fe8962003f51fd916204220205d8f201ac10100\n\n2016.08.18 17:13:08.163 ble_evt_attclient_attribute_value connection: 0 (0x00) atthandle: 15 (0x000f) type: 1 (0x01) value:02cdfe29fe58013dff4541aa0000000000000000\n2016.08.18 17:13:08.164 RX: 80190405000f00011402cdfe29fe58013dff4541aa0000000000000000\n\n2016.08.18 17:13:08.261 ble_evt_attclient_attribute_value connection: 0 (0x00) atthandle: 11 (0x000b) type: 1 (0x01) value:1fe8972003f71fd917204222205d90201ac10100\n2016.08.18 17:13:08.262 RX: 80190405000b0001141fe8972003f71fd917204222205d90201ac10100\n\n2016.08.18 17:13:08.263 ble_evt_attclient_attribute_value connection: 0 (0x00) atthandle: 15 (0x000f) type: 1 (0x01) value:02bafe2afe550139ff4141b20000000000000000\n2016.08.18 17:13:08.265 RX: 80190405000f00011402bafe2afe550139ff4141b20000000000000000\n\n2016.08.18 17:13:08.358 ble_evt_attclient_attribute_value connection: 0 (0x00) atthandle: 11 (0x000b) type: 1 (0x01) value:1fe8922003f41fd91820421d205d8d201abd0100\n2016.08.18 17:13:08.360 RX: 80190405000b0001141fe8922003f41fd91820421d205d8d201abd0100\n\n2016.08.18 17:13:08.361 ble_evt_attclient_attribute_value connection: 0 (0x00) atthandle: 15 (0x000f) type: 1 (0x01) value:02b6fe2cfe520142ff3141b90000000000000000\n2016.08.18 17:13:08.362 RX: 80190405000f00011402b6fe2cfe520142ff3141b90000000000000000\n\n2016.08.18 17:13:08.456 ble_evt_attclient_attribute_value connection: 0 (0x00) atthandle: 11 (0x000b) type: 1 (0x01) value:1fe89e2003f41fd91e20421d205d96201ab90100\n2016.08.18 17:13:08.457 RX: 80190405000b0001141fe89e2003f41fd91e20421d205d96201ab90100\n\n2016.08.18 17:13:08.458 ble_evt_attclient_attribute_value connection: 0 (0x00) atthandle: 15 (0x000f) type: 1 (0x01) value:02bafe34fe51014bff3441b80000000000000000\n2016.08.18 17:13:08.460 RX: 80190405000f00011402bafe34fe51014bff3441b80000000000000000\n\n2016.08.18 17:13:08.561 ble_evt_attclient_attribute_value connection: 0 (0x00) atthandle: 11 (0x000b) type: 1 (0x01) value:1fe89c2003f51fd91b20421c205d90201ab50100\n2016.08.18 17:13:08.562 RX: 80190405000b0001141fe89c2003f51fd91b20421c205d90201ab50100\n\n2016.08.18 17:13:08.563 ble_evt_attclient_attribute_value connection: 0 (0x00) atthandle: 15 (0x000f) type: 1 (0x01) value:02befe2dfe3c014fff4241ba0000000000000000\n2016.08.18 17:13:08.565 RX: 80190405000f00011402befe2dfe3c014fff4241ba0000000000000000\n\n2016.08.18 17:13:08.658 ble_evt_attclient_attribute_value connection: 0 (0x00) atthandle: 11 (0x000b) type: 1 (0x01) value:1fe89f2003f11fd91a204220205d8f201ab50100\n2016.08.18 17:13:08.660 RX: 80190405000b0001141fe89f2003f11fd91a204220205d8f201ab50100\n\n2016.08.18 17:13:08.661 ble_evt_attclient_attribute_value connection: 0 (0x00) atthandle: 15 (0x000f) type: 1 (0x01) value:02befe2cfe44014bff5641c60000000000000000\n2016.08.18 17:13:08.662 RX: 80190405000f00011402befe2cfe44014bff5641c60000000000000000\n\n2016.08.18 17:13:08.756 ble_evt_attclient_attribute_value connection: 0 (0x00) atthandle: 11 (0x000b) type: 1 (0x01) value:1fe89d2003f21fd91a204222205d8b201ab40100\n2016.08.18 17:13:08.757 RX: 80190405000b0001141fe89d2003f21fd91a204222205d8b201ab40100\n\n2016.08.18 17:13:08.758 ble_evt_attclient_attribute_value connection: 0 (0x00) atthandle: 15 (0x000f) type: 1 (0x01) value:02bbfe29fe4a012dff5041bb0000000000000000\n2016.08.18 17:13:08.760 RX: 80190405000f00011402bbfe29fe4a012dff5041bb0000000000000000\n\n2016.08.18 17:13:08.861 ble_evt_attclient_attribute_value connection: 0 (0x00) atthandle: 11 (0x000b) type: 1 (0x01) value:1fe89c2003f01fd918204221205d8a201ab00100\n2016.08.18 17:13:08.861 RX: 80190405000b0001141fe89c2003f01fd918204221205d8a201ab00100\n\n2016.08.18 17:13:08.863 ble_evt_attclient_attribute_value connection: 0 (0x00) atthandle: 15 (0x000f) type: 1 (0x01) value:02c3fe2efe4a0138ff4041bf0000000000000000\n2016.08.18 17:13:08.863 RX: 80190405000f00011402c3fe2efe4a0138ff4041bf0000000000000000\n\n2016.08.18 17:13:08.958 ble_evt_attclient_attribute_value connection: 0 (0x00) atthandle: 11 (0x000b) type: 1 (0x01) value:1fe89c2003f71fd91720422a205d92201ab30100\n2016.08.18 17:13:08.960 RX: 80190405000b0001141fe89c2003f71fd91720422a205d92201ab30100\n\n2016.08.18 17:13:08.961 ble_evt_attclient_attribute_value connection: 0 (0x00) atthandle: 15 (0x000f) type: 1 (0x01) value:02c4fe23fe420155ff2d41c40000000000000000\n2016.08.18 17:13:08.962 RX: 80190405000f00011402c4fe23fe420155ff2d41c40000000000000000\n\n2016.08.18 17:13:09.056 ble_evt_attclient_attribute_value connection: 0 (0x00) atthandle: 11 (0x000b) type: 1 (0x01) value:1fe89e2003fe1fd91a20422d205d99201abf0100\n2016.08.18 17:13:09.057 RX: 80190405000b0001141fe89e2003fe1fd91a20422d205d99201abf0100\n\n2016.08.18 17:13:09.058 ble_evt_attclient_attribute_value connection: 0 (0x00) atthandle: 15 (0x000f) type: 1 (0x01) value:02bdfe2dfe4e0150ff3c41be0000000000000000\n2016.08.18 17:13:09.060 RX: 80190405000f00011402bdfe2dfe4e0150ff3c41be0000000000000000\n\n2016.08.18 17:13:09.161 ble_evt_attclient_attribute_value connection: 0 (0x00) atthandle: 11 (0x000b) type: 1 (0x01) value:1fe8a12003fb1fd91d20422e205d9c201ac30100\n2016.08.18 17:13:09.162 RX: 80190405000b0001141fe8a12003fb1fd91d20422e205d9c201ac30100\n\n2016.08.18 17:13:09.163 ble_evt_attclient_attribute_value connection: 0 (0x00) atthandle: 15 (0x000f) type: 1 (0x01) value:02cbfe26fe47014dff4041b60000000000000000\n2016.08.18 17:13:09.165 RX: 80190405000f00011402cbfe26fe47014dff4041b60000000000000000\n\n2016.08.18 17:13:09.258 ble_evt_attclient_attribute_value connection: 0 (0x00) atthandle: 11 (0x000b) type: 1 (0x01) value:1fe89f2003fc1fd91b20422e205d9b201ac00100\n2016.08.18 17:13:09.260 RX: 80190405000b0001141fe89f2003fc1fd91b20422e205d9b201ac00100\n\n2016.08.18 17:13:09.261 ble_evt_attclient_attribute_value connection: 0 (0x00) atthandle: 15 (0x000f) type: 1 (0x01) value:02b7fe2ffe520149ff4d41c30000000000000000\n2016.08.18 17:13:09.262 RX: 80190405000f00011402b7fe2ffe520149ff4d41c30000000000000000\n\n2016.08.18 17:13:09.356 ble_evt_attclient_attribute_value connection: 0 (0x00) atthandle: 11 (0x000b) type: 1 (0x01) value:1fe89c2003fc1fd917204228205d92201ab90100\n2016.08.18 17:13:09.357 RX: 80190405000b0001141fe89c2003fc1fd917204228205d92201ab90100\n\n2016.08.18 17:13:09.359 ble_evt_attclient_attribute_value connection: 0 (0x00) atthandle: 15 (0x000f) type: 1 (0x01) value:02c5fe34fe50013fff3841ae0000000000000000\n2016.08.18 17:13:09.360 RX: 80190405000f00011402c5fe34fe50013fff3841ae0000000000000000\n\n2016.08.18 17:13:09.461 ble_evt_attclient_attribute_value connection: 0 (0x00) atthandle: 11 (0x000b) type: 1 (0x01) value:1fe8982003fd1fd916204227205d92201abe0100\n2016.08.18 17:13:09.462 RX: 80190405000b0001141fe8982003fd1fd916204227205d92201abe0100\n\n2016.08.18 17:13:09.463 ble_evt_attclient_attribute_value connection: 0 (0x00) atthandle: 15 (0x000f) type: 1 (0x01) value:02affe3cfe56015dff2441a40000000000000000\n2016.08.18 17:13:09.465 RX: 80190405000f00011402affe3cfe56015dff2441a40000000000000000\n\n2016.08.18 17:13:09.558 ble_evt_attclient_attribute_value connection: 0 (0x00) atthandle: 11 (0x000b) type: 1 (0x01) value:1fe89c2003fe1fd919204225205d98201aba0100\n2016.08.18 17:13:09.560 RX: 80190405000b0001141fe89c2003fe1fd919204225205d98201aba0100\n\n2016.08.18 17:13:09.561 ble_evt_attclient_attribute_value connection: 0 (0x00) atthandle: 15 (0x000f) type: 1 (0x01) value:02bbfe22fe4e016bff2441c60000000000000000\n2016.08.18 17:13:09.562 RX: 80190405000f00011402bbfe22fe4e016bff2441c60000000000000000\n\n2016.08.18 17:13:09.656 ble_evt_attclient_attribute_value connection: 0 (0x00) atthandle: 11 (0x000b) type: 1 (0x01) value:1fe89a2003f91fd91b204228205d98201aba0100\n2016.08.18 17:13:09.657 RX: 80190405000b0001141fe89a2003f91fd91b204228205d98201aba0100\n\n2016.08.18 17:13:09.658 ble_evt_attclient_attribute_value connection: 0 (0x00) atthandle: 15 (0x000f) type: 1 (0x01) value:02c3fe27fe470180ff4d41d10000000000000000\n2016.08.18 17:13:09.660 RX: 80190405000f00011402c3fe27fe470180ff4d41d10000000000000000\n\n2016.08.18 17:13:09.761 ble_evt_attclient_attribute_value connection: 0 (0x00) atthandle: 11 (0x000b) type: 1 (0x01) value:1fe8952003f51fd91820421f205d93201ab60100\n2016.08.18 17:13:09.762 RX: 80190405000b0001141fe8952003f51fd91820421f205d93201ab60100\n\n2016.08.18 17:13:09.763 ble_evt_attclient_attribute_value connection: 0 (0x00) atthandle: 15 (0x000f) type: 1 (0x01) value:02c6fe26fe4b013eff5141c90000000000000000\n2016.08.18 17:13:09.765 RX: 80190405000f00011402c6fe26fe4b013eff5141c90000000000000000\n\n2016.08.18 17:13:09.858 ble_evt_attclient_attribute_value connection: 0 (0x00) atthandle: 11 (0x000b) type: 1 (0x01) value:1fe8922003f11fd91820421d205d93201ab10100\n2016.08.18 17:13:09.860 RX: 80190405000b0001141fe8922003f11fd91820421d205d93201ab10100\n\n2016.08.18 17:13:09.861 ble_evt_attclient_attribute_value connection: 0 (0x00) atthandle: 15 (0x000f) type: 1 (0x01) value:02b0fe31fe4e0136ff4e41b50000000000000000\n2016.08.18 17:13:09.862 RX: 80190405000f00011402b0fe31fe4e0136ff4e41b50000000000000000\n\n2016.08.18 17:13:09.956 ble_evt_attclient_attribute_value connection: 0 (0x00) atthandle: 11 (0x000b) type: 1 (0x01) value:1fe88f2003e91fd912204219205d8e201aae0100\n2016.08.18 17:13:09.957 RX: 80190405000b0001141fe88f2003e91fd912204219205d8e201aae0100\n\n2016.08.18 17:13:09.958 ble_evt_attclient_attribute_value connection: 0 (0x00) atthandle: 15 (0x000f) type: 1 (0x01) value:02c3fe29fe520145ff1c418f0000000000000000\n2016.08.18 17:13:09.960 RX: 80190405000f00011402c3fe29fe520145ff1c418f0000000000000000\n\n2016.08.18 17:13:10.061 ble_evt_attclient_attribute_value connection: 0 (0x00) atthandle: 11 (0x000b) type: 1 (0x01) value:1fe88f2003ea1fd913204218205d8e201ab00100\n2016.08.18 17:13:10.062 RX: 80190405000b0001141fe88f2003ea1fd913204218205d8e201ab00100\n\n2016.08.18 17:13:10.063 ble_evt_attclient_attribute_value connection: 0 (0x00) atthandle: 15 (0x000f) type: 1 (0x01) value:02c0fe2afe52015dff3141a30000000000000000\n2016.08.18 17:13:10.065 RX: 80190405000f00011402c0fe2afe52015dff3141a30000000000000000\n\n2016.08.18 17:13:10.166 ble_evt_attclient_attribute_value connection: 0 (0x00) atthandle: 11 (0x000b) type: 1 (0x01) value:1fe8932003ec1fd91320421a205d8e201ab00100\n2016.08.18 17:13:10.167 RX: 80190405000b0001141fe8932003ec1fd91320421a205d8e201ab00100\n\n2016.08.18 17:13:10.168 ble_evt_attclient_attribute_value connection: 0 (0x00) atthandle: 15 (0x000f) type: 1 (0x01) value:02c8fe28fe4a0176ff4341ba0000000000000000\n2016.08.18 17:13:10.170 RX: 80190405000f00011402c8fe28fe4a0176ff4341ba0000000000000000\n\n2016.08.18 17:13:10.256 ble_evt_attclient_attribute_value connection: 0 (0x00) atthandle: 11 (0x000b) type: 1 (0x01) value:1fe8892003ee1fd914204219205d92201aae0100\n2016.08.18 17:13:10.257 RX: 80190405000b0001141fe8892003ee1fd914204219205d92201aae0100\n\n2016.08.18 17:13:10.258 ble_evt_attclient_attribute_value connection: 0 (0x00) atthandle: 15 (0x000f) type: 1 (0x01) value:02b6fe29fe480139ff5a41b40000000000000000\n2016.08.18 17:13:10.260 RX: 80190405000f00011402b6fe29fe480139ff5a41b40000000000000000\n\n2016.08.18 17:13:10.368 ble_evt_attclient_attribute_value connection: 0 (0x00) atthandle: 11 (0x000b) type: 1 (0x01) value:1fe88c2003f01fd914204216205d97201ab20100\n2016.08.18 17:13:10.370 RX: 80190405000b0001141fe88c2003f01fd914204216205d97201ab20100\n\n2016.08.18 17:13:10.371 ble_evt_attclient_attribute_value connection: 0 (0x00) atthandle: 15 (0x000f) type: 1 (0x01) value:02b4fe2cfe590142ff4e41b50000000000000000\n2016.08.18 17:13:10.372 RX: 80190405000f00011402b4fe2cfe590142ff4e41b50000000000000000\n\n2016.08.18 17:13:10.458 ble_evt_attclient_attribute_value connection: 0 (0x00) atthandle: 11 (0x000b) type: 1 (0x01) value:1fe8912003f31fd91a20421a205d9c201ab50100\n2016.08.18 17:13:10.460 RX: 80190405000b0001141fe8912003f31fd91a20421a205d9c201ab50100\n\n2016.08.18 17:13:10.461 ble_evt_attclient_attribute_value connection: 0 (0x00) atthandle: 15 (0x000f) type: 1 (0x01) value:02cefe2ffe480153ff4541a10000000000000000\n2016.08.18 17:13:10.462 RX: 80190405000f00011402cefe2ffe480153ff4541a10000000000000000\n\n2016.08.18 17:13:10.556 ble_evt_attclient_attribute_value connection: 0 (0x00) atthandle: 11 (0x000b) type: 1 (0x01) value:1fe8982003fb1fd91d20421c205d9e201abb0100\n2016.08.18 17:13:10.557 RX: 80190405000b0001141fe8982003fb1fd91d20421c205d9e201abb0100\n\n2016.08.18 17:13:10.558 ble_evt_attclient_attribute_value connection: 0 (0x00) atthandle: 15 (0x000f) type: 1 (0x01) value:02d5fe2dfe47014aff3441980000000000000000\n2016.08.18 17:13:10.560 RX: 80190405000f00011402d5fe2dfe47014aff3441980000000000000000\n\n2016.08.18 17:13:10.661 ble_evt_attclient_attribute_value connection: 0 (0x00) atthandle: 11 (0x000b) type: 1 (0x01) value:1fe89a2003fc1fd91f20421b205d9d201abb0100\n2016.08.18 17:13:10.662 RX: 80190405000b0001141fe89a2003fc1fd91f20421b205d9d201abb0100\n\n2016.08.18 17:13:10.664 ble_evt_attclient_attribute_value connection: 0 (0x00) atthandle: 15 (0x000f) type: 1 (0x01) value:02c2fe2efe50015dff3441bf0000000000000000\n2016.08.18 17:13:10.665 RX: 80190405000f00011402c2fe2efe50015dff3441bf0000000000000000\n\n2016.08.18 17:13:10.758 ble_evt_attclient_attribute_value connection: 0 (0x00) atthandle: 11 (0x000b) type: 1 (0x01) value:1fe8952003fc1fd91c20421a205da0201abc0100\n2016.08.18 17:13:10.760 RX: 80190405000b0001141fe8952003fc1fd91c20421a205da0201abc0100\n\n2016.08.18 17:13:10.761 ble_evt_attclient_attribute_value connection: 0 (0x00) atthandle: 15 (0x000f) type: 1 (0x01) value:02cefe2ffe4a0163ff4541900000000000000000\n2016.08.18 17:13:10.762 RX: 80190405000f00011402cefe2ffe4a0163ff4541900000000000000000\n\n2016.08.18 17:13:10.855 ble_evt_attclient_attribute_value connection: 0 (0x00) atthandle: 11 (0x000b) type: 1 (0x01) value:1fe89a2004011fd92320421f205da2201aba0100\n2016.08.18 17:13:10.857 RX: 80190405000b0001141fe89a2004011fd92320421f205da2201aba0100\n\n2016.08.18 17:13:10.870 ble_evt_attclient_attribute_value connection: 0 (0x00) atthandle: 15 (0x000f) type: 1 (0x01) value:02d4fe23fe4a0133ff5241ad0000000000000000\n2016.08.18 17:13:10.871 RX: 80190405000f00011402d4fe23fe4a0133ff5241ad0000000000000000\n\n2016.08.18 17:13:10.961 ble_evt_attclient_attribute_value connection: 0 (0x00) atthandle: 11 (0x000b) type: 1 (0x01) value:1fe8952003fc1fd91a20421c205d97201ab20100\n2016.08.18 17:13:10.962 RX: 80190405000b0001141fe8952003fc1fd91a20421c205d97201ab20100\n\n2016.08.18 17:13:10.963 ble_evt_attclient_attribute_value connection: 0 (0x00) atthandle: 15 (0x000f) type: 1 (0x01) value:02c9fe2bfe470135ff7341c40000000000000000\n2016.08.18 17:13:10.964 RX: 80190405000f00011402c9fe2bfe470135ff7341c40000000000000000\n\n2016.08.18 17:13:11.058 ble_evt_attclient_attribute_value connection: 0 (0x00) atthandle: 11 (0x000b) type: 1 (0x01) value:1fe8972003fd1fd91720421b205d95201ab20100\n2016.08.18 17:13:11.060 RX: 80190405000b0001141fe8972003fd1fd91720421b205d95201ab20100\n\n2016.08.18 17:13:11.061 ble_evt_attclient_attribute_value connection: 0 (0x00) atthandle: 15 (0x000f) type: 1 (0x01) value:02d5fe26fe4b012dff3641bf0000000000000000\n2016.08.18 17:13:11.062 RX: 80190405000f00011402d5fe26fe4b012dff3641bf0000000000000000\n\n2016.08.18 17:13:11.156 ble_evt_attclient_attribute_value connection: 0 (0x00) atthandle: 11 (0x000b) type: 1 (0x01) value:1fe8972003fd1fd91420421b205d95201ab10100\n2016.08.18 17:13:11.157 RX: 80190405000b0001141fe8972003fd1fd91420421b205d95201ab10100\n\n2016.08.18 17:13:11.158 ble_evt_attclient_attribute_value connection: 0 (0x00) atthandle: 15 (0x000f) type: 1 (0x01) value:02c4fe29fe480163ff1641aa0000000000000000\n2016.08.18 17:13:11.160 RX: 80190405000f00011402c4fe29fe480163ff1641aa0000000000000000\n\n2016.08.18 17:13:11.261 ble_evt_attclient_attribute_value connection: 0 (0x00) atthandle: 11 (0x000b) type: 1 (0x01) value:1fe8982003fc1fd91420421b205d91201abf0100\n2016.08.18 17:13:11.262 RX: 80190405000b0001141fe8982003fc1fd91420421b205d91201abf0100\n\n2016.08.18 17:13:11.263 ble_evt_attclient_attribute_value connection: 0 (0x00) atthandle: 15 (0x000f) type: 1 (0x01) value:02c1fe32fe490171ff38419b0000000000000000\n2016.08.18 17:13:11.265 RX: 80190405000f00011402c1fe32fe490171ff38419b0000000000000000\n\n2016.08.18 17:13:11.358 ble_evt_attclient_attribute_value connection: 0 (0x00) atthandle: 11 (0x000b) type: 1 (0x01) value:1fe8992003f91fd91420421b205d91201ac40100\n2016.08.18 17:13:11.360 RX: 80190405000b0001141fe8992003f91fd91420421b205d91201ac40100\n\n2016.08.18 17:13:11.361 ble_evt_attclient_attribute_value connection: 0 (0x00) atthandle: 15 (0x000f) type: 1 (0x01) value:02bcfe31fe500150ff4741b70000000000000000\n2016.08.18 17:13:11.362 RX: 80190405000f00011402bcfe31fe500150ff4741b70000000000000000\n\n2016.08.18 17:13:11.456 ble_evt_attclient_attribute_value connection: 0 (0x00) atthandle: 11 (0x000b) type: 1 (0x01) value:1fe8982003f71fd911204223205d8f201ac40100\n2016.08.18 17:13:11.457 RX: 80190405000b0001141fe8982003f71fd911204223205d8f201ac40100\n\n2016.08.18 17:13:11.458 ble_evt_attclient_attribute_value connection: 0 (0x00) atthandle: 15 (0x000f) type: 1 (0x01) value:02c6fe21fe480144ff5341bc0000000000000000\n2016.08.18 17:13:11.460 RX: 80190405000f00011402c6fe21fe480144ff5341bc0000000000000000\n\n2016.08.18 17:13:11.561 ble_evt_attclient_attribute_value connection: 0 (0x00) atthandle: 11 (0x000b) type: 1 (0x01) value:1fe89e2003f81fd914204224205d93201ac00100\n2016.08.18 17:13:11.562 RX: 80190405000b0001141fe89e2003f81fd914204224205d93201ac00100\n\n2016.08.18 17:13:11.563 ble_evt_attclient_attribute_value connection: 0 (0x00) atthandle: 15 (0x000f) type: 1 (0x01) value:02cafe27fe3c0135ff4941c20000000000000000\n2016.08.18 17:13:11.565 RX: 80190405000f00011402cafe27fe3c0135ff4941c20000000000000000\n\n2016.08.18 17:13:11.658 ble_evt_attclient_attribute_value connection: 0 (0x00) atthandle: 11 (0x000b) type: 1 (0x01) value:1fe89c2003f91fd916204227205d91201ac20100\n2016.08.18 17:13:11.660 RX: 80190405000b0001141fe89c2003f91fd916204227205d91201ac20100\n\n2016.08.18 17:13:11.661 ble_evt_attclient_attribute_value connection: 0 (0x00) atthandle: 15 (0x000f) type: 1 (0x01) value:02c1fe2dfe4b013aff3941aa0000000000000000\n2016.08.18 17:13:11.662 RX: 80190405000f00011402c1fe2dfe4b013aff3941aa0000000000000000\n\n2016.08.18 17:13:11.756 ble_evt_attclient_attribute_value connection: 0 (0x00) atthandle: 11 (0x000b) type: 1 (0x01) value:1fe8992003fc1fd915204223205d91201ac40100\n2016.08.18 17:13:11.757 RX: 80190405000b0001141fe8992003fc1fd915204223205d91201ac40100\n\n2016.08.18 17:13:11.758 ble_evt_attclient_attribute_value connection: 0 (0x00) atthandle: 15 (0x000f) type: 1 (0x01) value:02bbfe2bfe40015aff3141c10000000000000000\n2016.08.18 17:13:11.760 RX: 80190405000f00011402bbfe2bfe40015aff3141c10000000000000000\n\n2016.08.18 17:13:11.861 ble_evt_attclient_attribute_value connection: 0 (0x00) atthandle: 11 (0x000b) type: 1 (0x01) value:1fe89d2003fd1fd916204222205d8e201ac50100\n2016.08.18 17:13:11.862 RX: 80190405000b0001141fe89d2003fd1fd916204222205d8e201ac50100\n\n2016.08.18 17:13:11.863 ble_evt_attclient_attribute_value connection: 0 (0x00) atthandle: 15 (0x000f) type: 1 (0x01) value:02cefe28fe4d0163ff4441970000000000000000\n2016.08.18 17:13:11.864 RX: 80190405000f00011402cefe28fe4d0163ff4441970000000000000000\n\n2016.08.18 17:13:11.958 ble_evt_attclient_attribute_value connection: 0 (0x00) atthandle: 11 (0x000b) type: 1 (0x01) value:1fe89d2003fb1fd919204221205d91201ac60100\n2016.08.18 17:13:11.960 RX: 80190405000b0001141fe89d2003fb1fd919204221205d91201ac60100\n\n2016.08.18 17:13:11.961 ble_evt_attclient_attribute_value connection: 0 (0x00) atthandle: 15 (0x000f) type: 1 (0x01) value:02bffe2afe48014aff4841be0000000000000000\n2016.08.18 17:13:11.962 RX: 80190405000f00011402bffe2afe48014aff4841be0000000000000000\n\n2016.08.18 17:13:12.055 ble_evt_attclient_attribute_value connection: 0 (0x00) atthandle: 11 (0x000b) type: 1 (0x01) value:1fe89c2003f71fd91e204222205d8f201ac10100\n2016.08.18 17:13:12.057 RX: 80190405000b0001141fe89c2003f71fd91e204222205d8f201ac10100\n\n2016.08.18 17:13:12.058 ble_evt_attclient_attribute_value connection: 0 (0x00) atthandle: 15 (0x000f) type: 1 (0x01) value:02bcfe22fe490140ff3f41af0000000000000000\n2016.08.18 17:13:12.059 RX: 80190405000f00011402bcfe22fe490140ff3f41af0000000000000000\n\n2016.08.18 17:13:12.161 ble_evt_attclient_attribute_value connection: 0 (0x00) atthandle: 11 (0x000b) type: 1 (0x01) value:1fe8a72003fe1fd922204224205d93201ac00100\n2016.08.18 17:13:12.162 RX: 80190405000b0001141fe8a72003fe1fd922204224205d93201ac00100\n\n2016.08.18 17:13:12.163 ble_evt_attclient_attribute_value connection: 0 (0x00) atthandle: 15 (0x000f) type: 1 (0x01) value:02bcfe2afe490145ff39419a0000000000000000\n2016.08.18 17:13:12.165 RX: 80190405000f00011402bcfe2afe490145ff39419a0000000000000000\n\n2016.08.18 17:13:12.258 ble_evt_attclient_attribute_value connection: 0 (0x00) atthandle: 11 (0x000b) type: 1 (0x01) value:1fe8a52003fd1fd91d204220205d8e201ab50100\n2016.08.18 17:13:12.260 RX: 80190405000b0001141fe8a52003fd1fd91d204220205d8e201ab50100\n\n2016.08.18 17:13:12.261 ble_evt_attclient_attribute_value connection: 0 (0x00) atthandle: 15 (0x000f) type: 1 (0x01) value:02bbfe2bfe4b0162ff2041a20000000000000000\n2016.08.18 17:13:12.262 RX: 80190405000f00011402bbfe2bfe4b0162ff2041a20000000000000000\n\n2016.08.18 17:13:12.355 ble_evt_attclient_attribute_value connection: 0 (0x00) atthandle: 11 (0x000b) type: 1 (0x01) value:1fe8a92003fc1fd91f204223205d8d201ab70100\n2016.08.18 17:13:12.357 RX: 80190405000b0001141fe8a92003fc1fd91f204223205d8d201ab70100\n\n2016.08.18 17:13:12.358 ble_evt_attclient_attribute_value connection: 0 (0x00) atthandle: 15 (0x000f) type: 1 (0x01) value:02c3fe32fe4a0150ff3b41ad0000000000000000\n2016.08.18 17:13:12.359 RX: 80190405000f00011402c3fe32fe4a0150ff3b41ad0000000000000000\n\n2016.08.18 17:13:12.460 ble_evt_attclient_attribute_value connection: 0 (0x00) atthandle: 11 (0x000b) type: 1 (0x01) value:1fe8a42003fc1fd91d204222205d89201ab30100\n2016.08.18 17:13:12.462 RX: 80190405000b0001141fe8a42003fc1fd91d204222205d89201ab30100\n\n2016.08.18 17:13:12.464 ble_evt_attclient_attribute_value connection: 0 (0x00) atthandle: 15 (0x000f) type: 1 (0x01) value:02c2fe24fe4f0151ff6141b60000000000000000\n2016.08.18 17:13:12.466 RX: 80190405000f00011402c2fe24fe4f0151ff6141b60000000000000000\n\n2016.08.18 17:13:12.558 ble_evt_attclient_attribute_value connection: 0 (0x00) atthandle: 11 (0x000b) type: 1 (0x01) value:1fe8a12003fd1fd91d204221205d8a201ab00100\n2016.08.18 17:13:12.560 RX: 80190405000b0001141fe8a12003fd1fd91d204221205d8a201ab00100\n\n2016.08.18 17:13:12.561 ble_evt_attclient_attribute_value connection: 0 (0x00) atthandle: 15 (0x000f) type: 1 (0x01) value:02c1fe31fe4d014cff5b41a60000000000000000\n2016.08.18 17:13:12.562 RX: 80190405000f00011402c1fe31fe4d014cff5b41a60000000000000000\n\n2016.08.18 17:13:12.655 ble_evt_attclient_attribute_value connection: 0 (0x00) atthandle: 11 (0x000b) type: 1 (0x01) value:1fe8a12003fe1fd91f204225205d8f201ab30100\n2016.08.18 17:13:12.657 RX: 80190405000b0001141fe8a12003fe1fd91f204225205d8f201ab30100\n\n2016.08.18 17:13:12.658 ble_evt_attclient_attribute_value connection: 0 (0x00) atthandle: 15 (0x000f) type: 1 (0x01) value:02b4fe28fe4a0150ff3d41b70000000000000000\n2016.08.18 17:13:12.660 RX: 80190405000f00011402b4fe28fe4a0150ff3d41b70000000000000000\n\n2016.08.18 17:13:12.761 ble_evt_attclient_attribute_value connection: 0 (0x00) atthandle: 11 (0x000b) type: 1 (0x01) value:1fe8a32004031fd91e20422b205d96201abb0100\n2016.08.18 17:13:12.762 RX: 80190405000b0001141fe8a32004031fd91e20422b205d96201abb0100\n\n2016.08.18 17:13:12.763 ble_evt_attclient_attribute_value connection: 0 (0x00) atthandle: 15 (0x000f) type: 1 (0x01) value:02c2fe29fe4f0131ff3641be0000000000000000\n2016.08.18 17:13:12.764 RX: 80190405000f00011402c2fe29fe4f0131ff3641be0000000000000000\n\n2016.08.18 17:13:12.858 ble_evt_attclient_attribute_value connection: 0 (0x00) atthandle: 11 (0x000b) type: 1 (0x01) value:1fe8a02004041fd91a20422b205d98201abf0100\n2016.08.18 17:13:12.859 RX: 80190405000b0001141fe8a02004041fd91a20422b205d98201abf0100\n\n2016.08.18 17:13:12.861 ble_evt_attclient_attribute_value connection: 0 (0x00) atthandle: 15 (0x000f) type: 1 (0x01) value:02c0fe2ffe4d0142ff2c41b10000000000000000\n2016.08.18 17:13:12.862 RX: 80190405000f00011402c0fe2ffe4d0142ff2c41b10000000000000000\n\n2016.08.18 17:13:12.955 ble_evt_attclient_attribute_value connection: 0 (0x00) atthandle: 11 (0x000b) type: 1 (0x01) value:1fe89f2004001fd915204227205d97201abb0100\n2016.08.18 17:13:12.957 RX: 80190405000b0001141fe89f2004001fd915204227205d97201abb0100\n\n2016.08.18 17:13:12.958 ble_evt_attclient_attribute_value connection: 0 (0x00) atthandle: 15 (0x000f) type: 1 (0x01) value:02c5fe2efe4a0164ff5041b10000000000000000\n2016.08.18 17:13:12.959 RX: 80190405000f00011402c5fe2efe4a0164ff5041b10000000000000000\n\n2016.08.18 17:13:13.060 ble_evt_attclient_attribute_value connection: 0 (0x00) atthandle: 11 (0x000b) type: 1 (0x01) value:1fe8972003ff1fd915204225205d90201ab90100\n2016.08.18 17:13:13.062 RX: 80190405000b0001141fe8972003ff1fd915204225205d90201ab90100\n\n2016.08.18 17:13:13.063 ble_evt_attclient_attribute_value connection: 0 (0x00) atthandle: 15 (0x000f) type: 1 (0x01) value:02c6fe2bfe4f014dff5c41aa0000000000000000\n2016.08.18 17:13:13.065 RX: 80190405000f00011402c6fe2bfe4f014dff5c41aa0000000000000000\n\n2016.08.18 17:13:13.158 ble_evt_attclient_attribute_value connection: 0 (0x00) atthandle: 11 (0x000b) type: 1 (0x01) value:1fe8962004011fd916204222205d92201abb0100\n2016.08.18 17:13:13.159 RX: 80190405000b0001141fe8962004011fd916204222205d92201abb0100\n\n2016.08.18 17:13:13.161 ble_evt_attclient_attribute_value connection: 0 (0x00) atthandle: 15 (0x000f) type: 1 (0x01) value:02c6fe28fe530140ff5841a50000000000000000\n2016.08.18 17:13:13.162 RX: 80190405000f00011402c6fe28fe530140ff5841a50000000000000000\n\n2016.08.18 17:13:13.255 ble_evt_attclient_attribute_value connection: 0 (0x00) atthandle: 11 (0x000b) type: 1 (0x01) value:1fe8982003ff1fd91620421e205d92201aba0100\n2016.08.18 17:13:13.257 RX: 80190405000b0001141fe8982003ff1fd91620421e205d92201aba0100\n\n2016.08.18 17:13:13.258 ble_evt_attclient_attribute_value connection: 0 (0x00) atthandle: 15 (0x000f) type: 1 (0x01) value:02c6fe2ffe4a0135ff4a41bf0000000000000000\n2016.08.18 17:13:13.259 RX: 80190405000f00011402c6fe2ffe4a0135ff4a41bf0000000000000000\n\n2016.08.18 17:13:13.360 ble_evt_attclient_attribute_value connection: 0 (0x00) atthandle: 11 (0x000b) type: 1 (0x01) value:1fe8992003fa1fd91b204228205d96201abb0100\n2016.08.18 17:13:13.362 RX: 80190405000b0001141fe8992003fa1fd91b204228205d96201abb0100\n\n2016.08.18 17:13:13.363 ble_evt_attclient_attribute_value connection: 0 (0x00) atthandle: 15 (0x000f) type: 1 (0x01) value:02c7fe28fe4e0158ff3a41a60000000000000000\n2016.08.18 17:13:13.364 RX: 80190405000f00011402c7fe28fe4e0158ff3a41a60000000000000000\n\n2016.08.18 17:13:13.458 ble_evt_attclient_attribute_value connection: 0 (0x00) atthandle: 11 (0x000b) type: 1 (0x01) value:1fe8992003f81fd918204223205d94201aba0100\n2016.08.18 17:13:13.459 RX: 80190405000b0001141fe8992003f81fd918204223205d94201aba0100\n\n2016.08.18 17:13:13.461 ble_evt_attclient_attribute_value connection: 0 (0x00) atthandle: 15 (0x000f) type: 1 (0x01) value:02c4fe24fe4a016bff17418e0000000000000000\n2016.08.18 17:13:13.462 RX: 80190405000f00011402c4fe24fe4a016bff17418e0000000000000000\n\n2016.08.18 17:13:13.556 ble_evt_attclient_attribute_value connection: 0 (0x00) atthandle: 11 (0x000b) type: 1 (0x01) value:1fe8982003f81fd918204221205d94201ab40100\n2016.08.18 17:13:13.557 RX: 80190405000b0001141fe8982003f81fd918204221205d94201ab40100\n\n2016.08.18 17:13:13.558 ble_evt_attclient_attribute_value connection: 0 (0x00) atthandle: 15 (0x000f) type: 1 (0x01) value:02b2fe2dfe550159ff3c419e0000000000000000\n2016.08.18 17:13:13.560 RX: 80190405000f00011402b2fe2dfe550159ff3c419e0000000000000000\n\n2016.08.18 17:13:13.660 ble_evt_attclient_attribute_value connection: 0 (0x00) atthandle: 11 (0x000b) type: 1 (0x01) value:1fe8952003f11fd915204221205d93201ab60100\n2016.08.18 17:13:13.662 RX: 80190405000b0001141fe8952003f11fd915204221205d93201ab60100\n\n2016.08.18 17:13:13.663 ble_evt_attclient_attribute_value connection: 0 (0x00) atthandle: 15 (0x000f) type: 1 (0x01) value:02bdfe2dfe480155ff6941b60000000000000000\n2016.08.18 17:13:13.664 RX: 80190405000f00011402bdfe2dfe480155ff6941b60000000000000000\n\n2016.08.18 17:13:13.758 ble_evt_attclient_attribute_value connection: 0 (0x00) atthandle: 11 (0x000b) type: 1 (0x01) value:1fe8902003ef1fd91620421e205d90201ab60100\n2016.08.18 17:13:13.759 RX: 80190405000b0001141fe8902003ef1fd91620421e205d90201ab60100\n\n2016.08.18 17:13:13.760 ble_evt_attclient_attribute_value connection: 0 (0x00) atthandle: 15 (0x000f) type: 1 (0x01) value:02bbfe34fe45012bff4841d10000000000000000\n2016.08.18 17:13:13.762 RX: 80190405000f00011402bbfe34fe45012bff4841d10000000000000000\n\n2016.08.18 17:13:13.855 ble_evt_attclient_attribute_value connection: 0 (0x00) atthandle: 11 (0x000b) type: 1 (0x01) value:1fe8902003f21fd914204221205d90201ab40100\n2016.08.18 17:13:13.857 RX: 80190405000b0001141fe8902003f21fd914204221205d90201ab40100\n\n2016.08.18 17:13:13.858 ble_evt_attclient_attribute_value connection: 0 (0x00) atthandle: 15 (0x000f) type: 1 (0x01) value:02b8fe1cfe510144ff3641af0000000000000000\n2016.08.18 17:13:13.859 RX: 80190405000f00011402b8fe1cfe510144ff3641af0000000000000000\n\n2016.08.18 17:13:13.960 ble_evt_attclient_attribute_value connection: 0 (0x00) atthandle: 11 (0x000b) type: 1 (0x01) value:1fe88b2003f41fd915204220205d92201ab30100\n2016.08.18 17:13:13.962 RX: 80190405000b0001141fe88b2003f41fd915204220205d92201ab30100\n\n2016.08.18 17:13:13.963 ble_evt_attclient_attribute_value connection: 0 (0x00) atthandle: 15 (0x000f) type: 1 (0x01) value:02b8fe2ffe560143ff4741930000000000000000\n2016.08.18 17:13:13.964 RX: 80190405000f00011402b8fe2ffe560143ff4741930000000000000000\n\n2016.08.18 17:13:14.058 ble_evt_attclient_attribute_value connection: 0 (0x00) atthandle: 11 (0x000b) type: 1 (0x01) value:1fe88b2003f11fd91320421d205d93201ab40100\n2016.08.18 17:13:14.058 RX: 80190405000b0001141fe88b2003f11fd91320421d205d93201ab40100\n\n2016.08.18 17:13:14.060 ble_evt_attclient_attribute_value connection: 0 (0x00) atthandle: 15 (0x000f) type: 1 (0x01) value:02b4fe2ffe520160ff33419b0000000000000000\n2016.08.18 17:13:14.061 RX: 80190405000f00011402b4fe2ffe520160ff33419b0000000000000000\n\n2016.08.18 17:13:14.155 ble_evt_attclient_attribute_value connection: 0 (0x00) atthandle: 11 (0x000b) type: 1 (0x01) value:1fe88b2003f51fd91920421f205d97201ab60100\n2016.08.18 17:13:14.157 RX: 80190405000b0001141fe88b2003f51fd91920421f205d97201ab60100\n\n2016.08.18 17:13:14.158 ble_evt_attclient_attribute_value connection: 0 (0x00) atthandle: 15 (0x000f) type: 1 (0x01) value:02b3fe2cfe4f0142ff6541cb0000000000000000\n2016.08.18 17:13:14.159 RX: 80190405000f00011402b3fe2cfe4f0142ff6541cb0000000000000000\n\n2016.08.18 17:13:14.260 ble_evt_attclient_attribute_value connection: 0 (0x00) atthandle: 11 (0x000b) type: 1 (0x01) value:1fe8922003f91fd91b20421d205d99201abd0100\n2016.08.18 17:13:14.262 RX: 80190405000b0001141fe8922003f91fd91b20421d205d99201abd0100\n\n2016.08.18 17:13:14.263 ble_evt_attclient_attribute_value connection: 0 (0x00) atthandle: 15 (0x000f) type: 1 (0x01) value:02c4fe2afe4c0147ff5b41b60000000000000000\n2016.08.18 17:13:14.264 RX: 80190405000f00011402c4fe2afe4c0147ff5b41b60000000000000000\n\n2016.08.18 17:13:14.358 ble_evt_attclient_attribute_value connection: 0 (0x00) atthandle: 11 (0x000b) type: 1 (0x01) value:1fe8942003fd1fd91f204223205d99201ac10100\n2016.08.18 17:13:14.359 RX: 80190405000b0001141fe8942003fd1fd91f204223205d99201ac10100\n\n2016.08.18 17:13:14.360 ble_evt_attclient_attribute_value connection: 0 (0x00) atthandle: 15 (0x000f) type: 1 (0x01) value:02b5fe2bfe530140ff2e41c00000000000000000\n2016.08.18 17:13:14.362 RX: 80190405000f00011402b5fe2bfe530140ff2e41c00000000000000000\n\n2016.08.18 17:13:14.456 ble_evt_attclient_attribute_value connection: 0 (0x00) atthandle: 11 (0x000b) type: 1 (0x01) value:1fe8932003fe1fd922204220205d9f201ac10100\n2016.08.18 17:13:14.457 RX: 80190405000b0001141fe8932003fe1fd922204220205d9f201ac10100\n\n2016.08.18 17:13:14.458 ble_evt_attclient_attribute_value connection: 0 (0x00) atthandle: 15 (0x000f) type: 1 (0x01) value:02c0fe24fe56014cff3a419f0000000000000000\n2016.08.18 17:13:14.459 RX: 80190405000f00011402c0fe24fe56014cff3a419f0000000000000000\n\n2016.08.18 17:13:14.560 ble_evt_attclient_attribute_value connection: 0 (0x00) atthandle: 11 (0x000b) type: 1 (0x01) value:1fe8942003ff1fd922204221205da1201ac00100\n2016.08.18 17:13:14.562 RX: 80190405000b0001141fe8942003ff1fd922204221205da1201ac00100\n\n2016.08.18 17:13:14.563 ble_evt_attclient_attribute_value connection: 0 (0x00) atthandle: 15 (0x000f) type: 1 (0x01) value:02cbfe2bfe43014cff3241b10000000000000000\n2016.08.18 17:13:14.564 RX: 80190405000f00011402cbfe2bfe43014cff3241b10000000000000000\n\n2016.08.18 17:13:14.658 ble_evt_attclient_attribute_value connection: 0 (0x00) atthandle: 11 (0x000b) type: 1 (0x01) value:1fe8982003fa1fd91f204221205d96201abb0100\n2016.08.18 17:13:14.659 RX: 80190405000b0001141fe8982003fa1fd91f204221205d96201abb0100\n\n2016.08.18 17:13:14.660 ble_evt_attclient_attribute_value connection: 0 (0x00) atthandle: 15 (0x000f) type: 1 (0x01) value:02c5fe2cfe520149ff4a41c10000000000000000\n2016.08.18 17:13:14.662 RX: 80190405000f00011402c5fe2cfe520149ff4a41c10000000000000000\n\n2016.08.18 17:13:14.756 ble_evt_attclient_attribute_value connection: 0 (0x00) atthandle: 11 (0x000b) type: 1 (0x01) value:1fe8952003f91fd91f204222205d99201ab90100\n2016.08.18 17:13:14.757 RX: 80190405000b0001141fe8952003f91fd91f204222205d99201ab90100\n\n2016.08.18 17:13:14.759 ble_evt_attclient_attribute_value connection: 0 (0x00) atthandle: 15 (0x000f) type: 1 (0x01) value:02bafe2bfe4c0147ff6741be0000000000000000\n2016.08.18 17:13:14.760 RX: 80190405000f00011402bafe2bfe4c0147ff6741be0000000000000000\n\n2016.08.18 17:13:14.860 ble_evt_attclient_attribute_value connection: 0 (0x00) atthandle: 11 (0x000b) type: 1 (0x01) value:1fe8942003f91fd91a20421e205d92201ab90100\n2016.08.18 17:13:14.862 RX: 80190405000b0001141fe8942003f91fd91a20421e205d92201ab90100\n\n2016.08.18 17:13:14.863 ble_evt_attclient_attribute_value connection: 0 (0x00) atthandle: 15 (0x000f) type: 1 (0x01) value:02cdfe2dfe470143ff4c41be0000000000000000\n2016.08.18 17:13:14.864 RX: 80190405000f00011402cdfe2dfe470143ff4c41be0000000000000000\n\n2016.08.18 17:13:14.958 ble_evt_attclient_attribute_value connection: 0 (0x00) atthandle: 11 (0x000b) type: 1 (0x01) value:1fe8922003f71fd919204216205d8d201abe0100\n2016.08.18 17:13:14.959 RX: 80190405000b0001141fe8922003f71fd919204216205d8d201abe0100\n\n2016.08.18 17:13:14.960 ble_evt_attclient_attribute_value connection: 0 (0x00) atthandle: 15 (0x000f) type: 1 (0x01) value:02bafe35fe4d013dff3e41a50000000000000000\n2016.08.18 17:13:14.962 RX: 80190405000f00011402bafe35fe4d013dff3e41a50000000000000000\n\n2016.08.18 17:13:15.055 ble_evt_attclient_attribute_value connection: 0 (0x00) atthandle: 11 (0x000b) type: 1 (0x01) value:1fe8902003f11fd917204218205d8c201abf0100\n2016.08.18 17:13:15.057 RX: 80190405000b0001141fe8902003f11fd917204218205d8c201abf0100\n\n2016.08.18 17:13:15.058 ble_evt_attclient_attribute_value connection: 0 (0x00) atthandle: 15 (0x000f) type: 1 (0x01) value:02c5fe26fe4c015cff2b41880000000000000000\n2016.08.18 17:13:15.059 RX: 80190405000f00011402c5fe26fe4c015cff2b41880000000000000000\n\n2016.08.18 17:13:15.160 ble_evt_attclient_attribute_value connection: 0 (0x00) atthandle: 11 (0x000b) type: 1 (0x01) value:1fe8972003f51fd919204222205d90201ac10100\n2016.08.18 17:13:15.162 RX: 80190405000b0001141fe8972003f51fd919204222205d90201ac10100\n\n2016.08.18 17:13:15.163 ble_evt_attclient_attribute_value connection: 0 (0x00) atthandle: 15 (0x000f) type: 1 (0x01) value:02b8fe2bfe4c0167ff3e41bd0000000000000000\n2016.08.18 17:13:15.164 RX: 80190405000f00011402b8fe2bfe4c0167ff3e41bd0000000000000000\n\n2016.08.18 17:13:15.258 ble_evt_attclient_attribute_value connection: 0 (0x00) atthandle: 11 (0x000b) type: 1 (0x01) value:1fe8972003f31fd919204222205d92201ac20100\n2016.08.18 17:13:15.259 RX: 80190405000b0001141fe8972003f31fd919204222205d92201ac20100\n\n2016.08.18 17:13:15.260 ble_evt_attclient_attribute_value connection: 0 (0x00) atthandle: 15 (0x000f) type: 1 (0x01) value:02c2fe27fe4d0150ff4341c20000000000000000\n2016.08.18 17:13:15.262 RX: 80190405000f00011402c2fe27fe4d0150ff4341c20000000000000000\n\n2016.08.18 17:13:15.355 ble_evt_attclient_attribute_value connection: 0 (0x00) atthandle: 11 (0x000b) type: 1 (0x01) value:1fe8982003f81fd91c204225205d94201abf0100\n2016.08.18 17:13:15.357 RX: 80190405000b0001141fe8982003f81fd91c204225205d94201abf0100\n\n2016.08.18 17:13:15.358 ble_evt_attclient_attribute_value connection: 0 (0x00) atthandle: 15 (0x000f) type: 1 (0x01) value:02bdfe2bfe4a0155ff5c41b10000000000000000\n2016.08.18 17:13:15.359 RX: 80190405000f00011402bdfe2bfe4a0155ff5c41b10000000000000000\n\n2016.08.18 17:13:15.460 ble_evt_attclient_attribute_value connection: 0 (0x00) atthandle: 11 (0x000b) type: 1 (0x01) value:1fe8912003f61fd91820421c205d8f201ab90100\n2016.08.18 17:13:15.462 RX: 80190405000b0001141fe8912003f61fd91820421c205d8f201ab90100\n\n2016.08.18 17:13:15.463 ble_evt_attclient_attribute_value connection: 0 (0x00) atthandle: 15 (0x000f) type: 1 (0x01) value:02c2fe29fe4e013eff4641a40000000000000000\n2016.08.18 17:13:15.464 RX: 80190405000f00011402c2fe29fe4e013eff4641a40000000000000000\n\n2016.08.18 17:13:15.558 ble_evt_attclient_attribute_value connection: 0 (0x00) atthandle: 11 (0x000b) type: 1 (0x01) value:1fe8902003f71fd91620421e205d8e201aba0100\n2016.08.18 17:13:15.559 RX: 80190405000b0001141fe8902003f71fd91620421e205d8e201aba0100\n\n2016.08.18 17:13:15.560 ble_evt_attclient_attribute_value connection: 0 (0x00) atthandle: 15 (0x000f) type: 1 (0x01) value:02bcfe28fe4f014eff3241cf0000000000000000\n2016.08.18 17:13:15.562 RX: 80190405000f00011402bcfe28fe4f014eff3241cf0000000000000000\n\n2016.08.18 17:13:15.655 ble_evt_attclient_attribute_value connection: 0 (0x00) atthandle: 11 (0x000b) type: 1 (0x01) value:1fe8912003f71fd91820421e205d89201aba0100\n2016.08.18 17:13:15.657 RX: 80190405000b0001141fe8912003f71fd91820421e205d89201aba0100\n\n2016.08.18 17:13:15.658 ble_evt_attclient_attribute_value connection: 0 (0x00) atthandle: 15 (0x000f) type: 1 (0x01) value:02cbfe29fe44016cff3041c20000000000000000\n2016.08.18 17:13:15.659 RX: 80190405000f00011402cbfe29fe44016cff3041c20000000000000000\n\n2016.08.18 17:13:15.760 ble_evt_attclient_attribute_value connection: 0 (0x00) atthandle: 11 (0x000b) type: 1 (0x01) value:1fe8902003f51fd91c20421d205d8a201ab90100\n2016.08.18 17:13:15.762 RX: 80190405000b0001141fe8902003f51fd91c20421d205d8a201ab90100\n\n2016.08.18 17:13:15.763 ble_evt_attclient_attribute_value connection: 0 (0x00) atthandle: 15 (0x000f) type: 1 (0x01) value:02c1fe22fe4b0153ff4e41b50000000000000000\n2016.08.18 17:13:15.764 RX: 80190405000f00011402c1fe22fe4b0153ff4e41b50000000000000000\n\n2016.08.18 17:13:15.858 ble_evt_attclient_attribute_value connection: 0 (0x00) atthandle: 11 (0x000b) type: 1 (0x01) value:1fe8902003f41fd92020421d205d8a201ab80100\n2016.08.18 17:13:15.859 RX: 80190405000b0001141fe8902003f41fd92020421d205d8a201ab80100\n\n2016.08.18 17:13:15.861 ble_evt_attclient_attribute_value connection: 0 (0x00) atthandle: 15 (0x000f) type: 1 (0x01) value:02c7fe28fe530157ff4741c00000000000000000\n2016.08.18 17:13:15.862 RX: 80190405000f00011402c7fe28fe530157ff4741c00000000000000000\n\n2016.08.18 17:13:15.955 ble_evt_attclient_attribute_value connection: 0 (0x00) atthandle: 11 (0x000b) type: 1 (0x01) value:1fe8972003f61fd91e20421d205d88201ab00100\n2016.08.18 17:13:15.957 RX: 80190405000b0001141fe8972003f61fd91e20421d205d88201ab00100\n\n2016.08.18 17:13:15.958 ble_evt_attclient_attribute_value connection: 0 (0x00) atthandle: 15 (0x000f) type: 1 (0x01) value:02c6fe21fe430139ff4441c40000000000000000\n2016.08.18 17:13:15.959 RX: 80190405000f00011402c6fe21fe430139ff4441c40000000000000000\n\n2016.08.18 17:13:16.060 ble_evt_attclient_attribute_value connection: 0 (0x00) atthandle: 11 (0x000b) type: 1 (0x01) value:1fe8982003f41fd91d204221205d89201ab10100\n2016.08.18 17:13:16.062 RX: 80190405000b0001141fe8982003f41fd91d204221205d89201ab10100\n\n2016.08.18 17:13:16.063 ble_evt_attclient_attribute_value connection: 0 (0x00) atthandle: 15 (0x000f) type: 1 (0x01) value:02bdfe23fe480148ff5241b10000000000000000\n2016.08.18 17:13:16.064 RX: 80190405000f00011402bdfe23fe480148ff5241b10000000000000000\n\n2016.08.18 17:13:16.158 ble_evt_attclient_attribute_value connection: 0 (0x00) atthandle: 11 (0x000b) type: 1 (0x01) value:1fe8972003ef1fd91c204221205d83201aab0100\n2016.08.18 17:13:16.159 RX: 80190405000b0001141fe8972003ef1fd91c204221205d83201aab0100\n\n2016.08.18 17:13:16.160 ble_evt_attclient_attribute_value connection: 0 (0x00) atthandle: 15 (0x000f) type: 1 (0x01) value:02c6fe29fe49014fff3241960000000000000000\n2016.08.18 17:13:16.162 RX: 80190405000f00011402c6fe29fe49014fff3241960000000000000000\n\n2016.08.18 17:13:16.255 ble_evt_attclient_attribute_value connection: 0 (0x00) atthandle: 11 (0x000b) type: 1 (0x01) value:1fe8982003ef1fd91a204222205d85201aa90100\n2016.08.18 17:13:16.257 RX: 80190405000b0001141fe8982003ef1fd91a204222205d85201aa90100\n\n2016.08.18 17:13:16.258 ble_evt_attclient_attribute_value connection: 0 (0x00) atthandle: 15 (0x000f) type: 1 (0x01) value:02bffe27fe51014fff1f41a70000000000000000\n2016.08.18 17:13:16.259 RX: 80190405000f00011402bffe27fe51014fff1f41a70000000000000000\n\n2016.08.18 17:13:16.360 ble_evt_attclient_attribute_value connection: 0 (0x00) atthandle: 11 (0x000b) type: 1 (0x01) value:1fe8942003ef1fd91a204220205d84201aa50100\n2016.08.18 17:13:16.362 RX: 80190405000b0001141fe8942003ef1fd91a204220205d84201aa50100\n\n2016.08.18 17:13:16.363 ble_evt_attclient_attribute_value connection: 0 (0x00) atthandle: 15 (0x000f) type: 1 (0x01) value:02c4fe29fe450155ff3a41960000000000000000\n2016.08.18 17:13:16.364 RX: 80190405000f00011402c4fe29fe450155ff3a41960000000000000000\n\n2016.08.18 17:13:16.458 ble_evt_attclient_attribute_value connection: 0 (0x00) atthandle: 11 (0x000b) type: 1 (0x01) value:1fe89a2003fa1fd91e20422c205d91201ab60100\n2016.08.18 17:13:16.459 RX: 80190405000b0001141fe89a2003fa1fd91e20422c205d91201ab60100\n\n2016.08.18 17:13:16.460 ble_evt_attclient_attribute_value connection: 0 (0x00) atthandle: 15 (0x000f) type: 1 (0x01) value:02b6fe2ffe420148ff4a41af0000000000000000\n2016.08.18 17:13:16.462 RX: 80190405000f00011402b6fe2ffe420148ff4a41af0000000000000000\n\n2016.08.18 17:13:16.555 ble_evt_attclient_attribute_value connection: 0 (0x00) atthandle: 11 (0x000b) type: 1 (0x01) value:1fe89d2003fb1fd92320422e205d97201aba0100\n2016.08.18 17:13:16.557 RX: 80190405000b0001141fe89d2003fb1fd92320422e205d97201aba0100\n\n2016.08.18 17:13:16.558 ble_evt_attclient_attribute_value connection: 0 (0x00) atthandle: 15 (0x000f) type: 1 (0x01) value:02bffe2afe49013cff5f41b90000000000000000\n2016.08.18 17:13:16.559 RX: 80190405000f00011402bffe2afe49013cff5f41b90000000000000000\n\n2016.08.18 17:13:16.660 ble_evt_attclient_attribute_value connection: 0 (0x00) atthandle: 11 (0x000b) type: 1 (0x01) value:1fe89a2003fa1fd91d204229205d93201ab90100\n2016.08.18 17:13:16.662 RX: 80190405000b0001141fe89a2003fa1fd91d204229205d93201ab90100\n\n2016.08.18 17:13:16.663 ble_evt_attclient_attribute_value connection: 0 (0x00) atthandle: 15 (0x000f) type: 1 (0x01) value:02bffe25fe44014fff4841ac0000000000000000\n2016.08.18 17:13:16.664 RX: 80190405000f00011402bffe25fe44014fff4841ac0000000000000000\n\n2016.08.18 17:13:16.758 ble_evt_attclient_attribute_value connection: 0 (0x00) atthandle: 11 (0x000b) type: 1 (0x01) value:1fe8932003f71fd918204220205d89201ab10100\n2016.08.18 17:13:16.759 RX: 80190405000b0001141fe8932003f71fd918204220205d89201ab10100\n\n2016.08.18 17:13:16.760 ble_evt_attclient_attribute_value connection: 0 (0x00) atthandle: 15 (0x000f) type: 1 (0x01) value:02bafe35fe4d0155ff2a41a20000000000000000\n2016.08.18 17:13:16.761 RX: 80190405000f00011402bafe35fe4d0155ff2a41a20000000000000000\n\n2016.08.18 17:13:16.855 ble_evt_attclient_attribute_value connection: 0 (0x00) atthandle: 11 (0x000b) type: 1 (0x01) value:1fe8922003fb1fd91c204224205d8c201ab30100\n2016.08.18 17:13:16.857 RX: 80190405000b0001141fe8922003fb1fd91c204224205d8c201ab30100\n\n2016.08.18 17:13:16.858 ble_evt_attclient_attribute_value connection: 0 (0x00) atthandle: 15 (0x000f) type: 1 (0x01) value:02c3fe24fe45016aff4041990000000000000000\n2016.08.18 17:13:16.859 RX: 80190405000f00011402c3fe24fe45016aff4041990000000000000000\n\n2016.08.18 17:13:16.960 ble_evt_attclient_attribute_value connection: 0 (0x00) atthandle: 11 (0x000b) type: 1 (0x01) value:1fe8952003fc1fd921204220205d90201ab70100\n2016.08.18 17:13:16.962 RX: 80190405000b0001141fe8952003fc1fd921204220205d90201ab70100\n\n2016.08.18 17:13:16.963 ble_evt_attclient_attribute_value connection: 0 (0x00) atthandle: 15 (0x000f) type: 1 (0x01) value:02c7fe29fe45013aff4441bd0000000000000000\n2016.08.18 17:13:16.964 RX: 80190405000f00011402c7fe29fe45013aff4441bd0000000000000000\n\n2016.08.18 17:13:17.058 ble_evt_attclient_attribute_value connection: 0 (0x00) atthandle: 11 (0x000b) type: 1 (0x01) value:1fe8922003fb1fd921204224205d8e201ab70100\n2016.08.18 17:13:17.059 RX: 80190405000b0001141fe8922003fb1fd921204224205d8e201ab70100\n\n2016.08.18 17:13:17.060 ble_evt_attclient_attribute_value connection: 0 (0x00) atthandle: 15 (0x000f) type: 1 (0x01) value:02bcfe2ffe4f0141ff4a41d20000000000000000\n2016.08.18 17:13:17.061 RX: 80190405000f00011402bcfe2ffe4f0141ff4a41d20000000000000000\n\n2016.08.18 17:13:17.155 ble_evt_attclient_attribute_value connection: 0 (0x00) atthandle: 11 (0x000b) type: 1 (0x01) value:1fe8932003fa1fd923204220205d8e201ab90100\n2016.08.18 17:13:17.157 RX: 80190405000b0001141fe8932003fa1fd923204220205d8e201ab90100\n\n2016.08.18 17:13:17.158 ble_evt_attclient_attribute_value connection: 0 (0x00) atthandle: 15 (0x000f) type: 1 (0x01) value:02cbfe27fe4c014aff3541d60000000000000000\n2016.08.18 17:13:17.160 RX: 80190405000f00011402cbfe27fe4c014aff3541d60000000000000000\n\n2016.08.18 17:13:17.260 ble_evt_attclient_attribute_value connection: 0 (0x00) atthandle: 11 (0x000b) type: 1 (0x01) value:1fe8902003f91fd92420421e205d92201ab70100\n2016.08.18 17:13:17.262 RX: 80190405000b0001141fe8902003f91fd92420421e205d92201ab70100\n\n2016.08.18 17:13:17.263 ble_evt_attclient_attribute_value connection: 0 (0x00) atthandle: 15 (0x000f) type: 1 (0x01) value:02bffe31fe550154ff3741960000000000000000\n2016.08.18 17:13:17.264 RX: 80190405000f00011402bffe31fe550154ff3741960000000000000000\n\n2016.08.18 17:13:17.358 ble_evt_attclient_attribute_value connection: 0 (0x00) atthandle: 11 (0x000b) type: 1 (0x01) value:1fe8902003f31fd92320421b205d8d201ab50100\n2016.08.18 17:13:17.359 RX: 80190405000b0001141fe8902003f31fd92320421b205d8d201ab50100\n\n2016.08.18 17:13:17.361 ble_evt_attclient_attribute_value connection: 0 (0x00) atthandle: 15 (0x000f) type: 1 (0x01) value:02c2fe2cfe4c015fff3741ad0000000000000000\n2016.08.18 17:13:17.362 RX: 80190405000f00011402c2fe2cfe4c015fff3741ad0000000000000000\n\n2016.08.18 17:13:17.455 ble_evt_attclient_attribute_value connection: 0 (0x00) atthandle: 11 (0x000b) type: 1 (0x01) value:1fe8902003f01fd91d204218205d8b201ab60100\n2016.08.18 17:13:17.457 RX: 80190405000b0001141fe8902003f01fd91d204218205d8b201ab60100\n\n2016.08.18 17:13:17.458 ble_evt_attclient_attribute_value connection: 0 (0x00) atthandle: 15 (0x000f) type: 1 (0x01) value:02ccfe25fe460157ff4f41a90000000000000000\n2016.08.18 17:13:17.459 RX: 80190405000f00011402ccfe25fe460157ff4f41a90000000000000000\n\n2016.08.18 17:13:17.560 ble_evt_attclient_attribute_value connection: 0 (0x00) atthandle: 11 (0x000b) type: 1 (0x01) value:1fe8952003f51fd92320421f205d8f201ab80100\n2016.08.18 17:13:17.562 RX: 80190405000b0001141fe8952003f51fd92320421f205d8f201ab80100\n\n2016.08.18 17:13:17.563 ble_evt_attclient_attribute_value connection: 0 (0x00) atthandle: 15 (0x000f) type: 1 (0x01) value:02bafe26fe440137ff5441e90000000000000000\n2016.08.18 17:13:17.565 RX: 80190405000f00011402bafe26fe440137ff5441e90000000000000000\n\n2016.08.18 17:13:17.658 ble_evt_attclient_attribute_value connection: 0 (0x00) atthandle: 11 (0x000b) type: 1 (0x01) value:1fe8922003f51fd92520421c205d90201ab40100\n2016.08.18 17:13:17.659 RX: 80190405000b0001141fe8922003f51fd92520421c205d90201ab40100\n\n2016.08.18 17:13:17.660 ble_evt_attclient_attribute_value connection: 0 (0x00) atthandle: 15 (0x000f) type: 1 (0x01) value:02c5fe25fe490140ff5541b40000000000000000\n2016.08.18 17:13:17.661 RX: 80190405000f00011402c5fe25fe490140ff5541b40000000000000000\n\n2016.08.18 17:13:17.755 ble_evt_attclient_attribute_value connection: 0 (0x00) atthandle: 11 (0x000b) type: 1 (0x01) value:1fe88f2003f51fd91c20421c205d93201ab50100\n2016.08.18 17:13:17.757 RX: 80190405000b0001141fe88f2003f51fd91c20421c205d93201ab50100\n\n2016.08.18 17:13:17.758 ble_evt_attclient_attribute_value connection: 0 (0x00) atthandle: 15 (0x000f) type: 1 (0x01) value:02cafe2ffe490145ff5941b50000000000000000\n2016.08.18 17:13:17.759 RX: 80190405000f00011402cafe2ffe490145ff5941b50000000000000000\n\n2016.08.18 17:13:17.860 ble_evt_attclient_attribute_value connection: 0 (0x00) atthandle: 11 (0x000b) type: 1 (0x01) value:1fe8902003f91fd92220421e205d99201aba0100\n2016.08.18 17:13:17.862 RX: 80190405000b0001141fe8902003f91fd92220421e205d99201aba0100\n\n2016.08.18 17:13:17.863 ble_evt_attclient_attribute_value connection: 0 (0x00) atthandle: 15 (0x000f) type: 1 (0x01) value:02c4fe1dfe470151ff3641900000000000000000\n2016.08.18 17:13:17.864 RX: 80190405000f00011402c4fe1dfe470151ff3641900000000000000000\n\n2016.08.18 17:13:17.957 ble_evt_attclient_attribute_value connection: 0 (0x00) atthandle: 11 (0x000b) type: 1 (0x01) value:1fe8992003fd1fd92520421c205d98201ac40100\n2016.08.18 17:13:17.959 RX: 80190405000b0001141fe8992003fd1fd92520421c205d98201ac40100\n\n2016.08.18 17:13:17.960 ble_evt_attclient_attribute_value connection: 0 (0x00) atthandle: 15 (0x000f) type: 1 (0x01) value:02c7fe32fe4e0163ff5841ad0000000000000000\n2016.08.18 17:13:17.961 RX: 80190405000f00011402c7fe32fe4e0163ff5841ad0000000000000000\n\n"
  # "Interval time Cal. from log data @ BLED112"
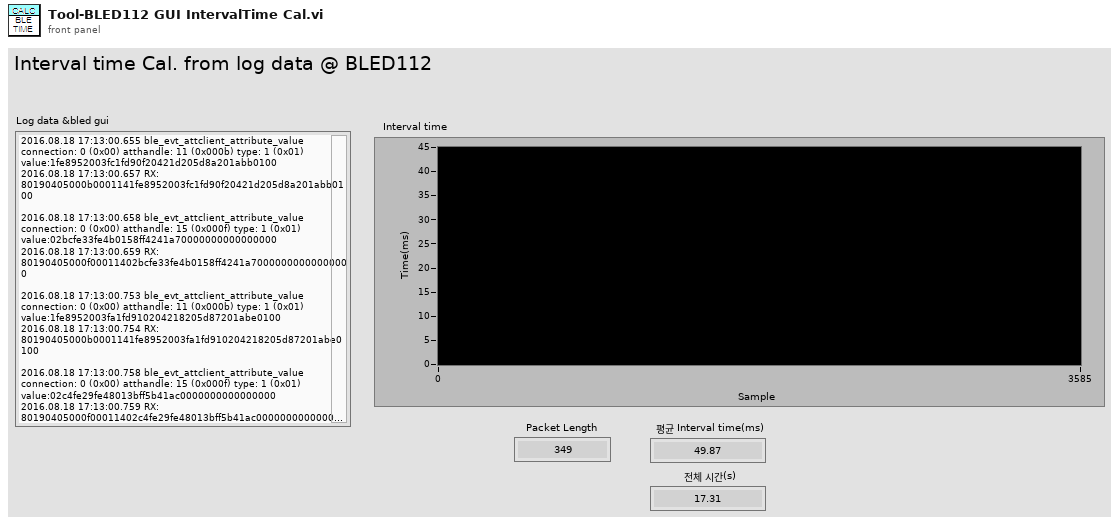
[diagram p1: front panel]
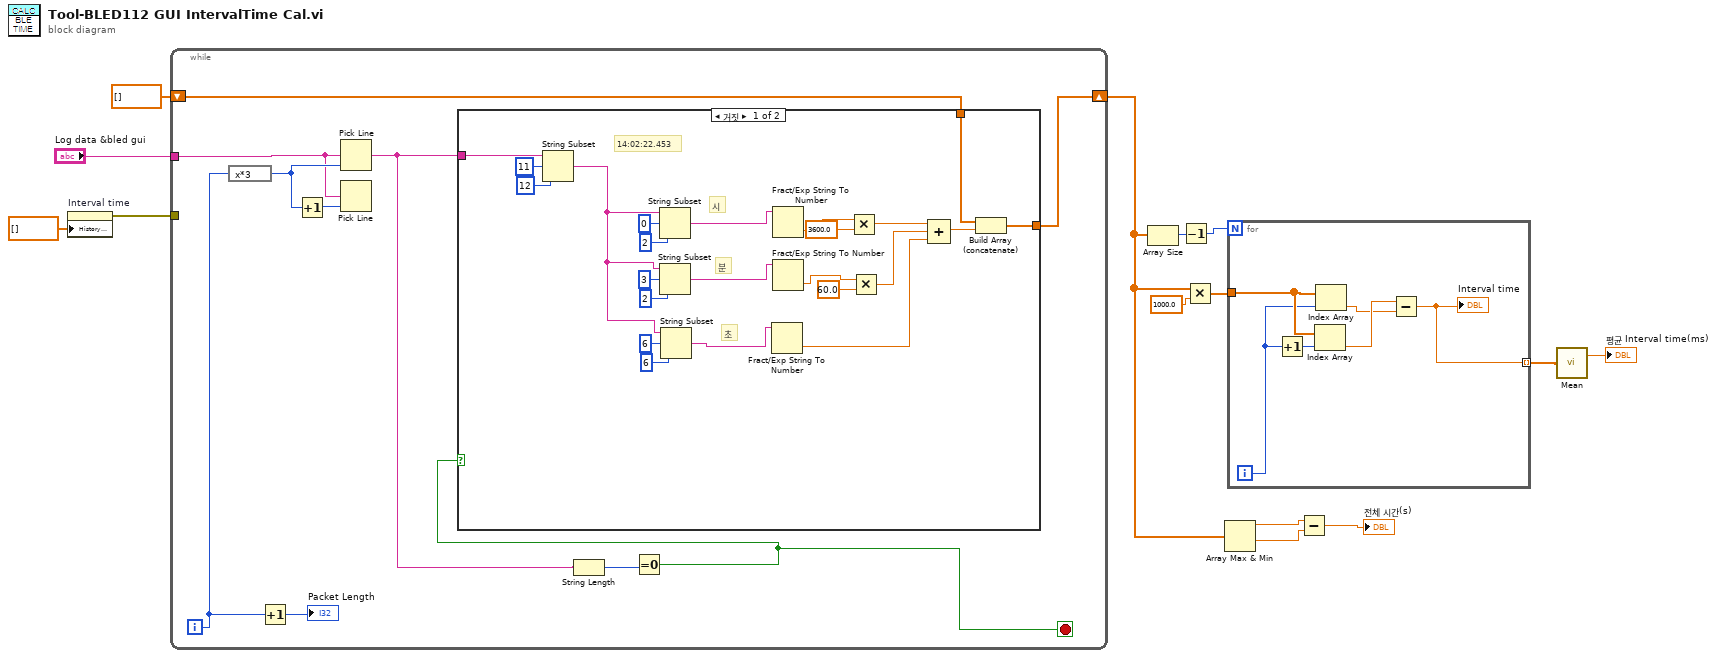
[diagram p0: block diagram]
diagram:
  n1 = property on="Interval time" class="WFChart (엄격한)"("History Data"=dbl[] [] ("히스토리 데이터")) -> (error out=w12:errorcluster)  [unwired: 2 in, 1 out]
  n2 = while {
    tunnel: "Log data &bled gui" -> [w22]
    tunnel: w12 -> [_]
    shift-right: [w20] -> w4
    shift-left: dbl[] [] -> [w21]
    i -> [w18]
    stop <- w17 stop-if-true
    n3 = expression code="x*3"(w18) -> (w24:i32)
    n4 = Increment(x=w18) -> (x+1=→"Packet Length":i32)
    n5 = Increment(x=w24) -> (x+1=w23:i32)
    n6 = Pick Line(multi-line string=w22, line index=w24) -> (output string=w16:string)  [unwired: 1 in]
    n7 = Pick Line(multi-line string=w22, line index=w23) -> ()  [unwired: 1 in, 1 out]
    n8 = String Length(string=w16) -> (length=w15:i32)
    n9 = Equal To 0?(x=w15) -> (x = 0?=w17:bool)
    n10 = case shown="거짓" w17 {
      tunnel: w16 -> [w47 _]
      tunnel: w21 -> [w27 w48]
      tunnel: [w25 w48] -> w20
      frame False {
        # "초"
        # "분"
        # "시"
        # "14:02:22.453"
        n11 = String Subset(string=w47, offset (0)=11 ("오프셋(0)"), length (rest)=12 ("길이(나머지)")) -> (substring=w38:string)
        n12 = String Subset(string=w38, offset (0)=0 ("오프셋(0)"), length (rest)=2 ("길이(나머지)")) -> (substring=w37:string)
        n13 = String Subset(string=w38, offset (0)=3 ("오프셋(0)"), length (rest)=2 ("길이(나머지)")) -> (substring=w36:string)
        n14 = String Subset(string=w38, offset (0)=6 ("오프셋(0)"), length (rest)=6 ("길이(나머지)")) -> (substring=w35:string)
        n15 = Fract/Exp String To Number(string=w35) -> (number=w28:dbl)  [unwired: 3 in, 1 out]
        n16 = Fract/Exp String To Number(string=w37) -> (number=w34:dbl)  [unwired: 3 in, 1 out]
        n17 = Fract/Exp String To Number(string=w36) -> (number=w31:dbl)  [unwired: 3 in, 1 out]
        n18 = Multiply(x=w34, y=3600.0) -> (x*y=w30:dbl)
        n19 = Multiply(x=w31, y=60.0) -> (x*y=w29:dbl)
        n20 = Compound Arithmetic op=ADD(w30, w29, w28) -> (w26:dbl)
        n21 = Build Array (concatenate)(w27, w26) -> (w25:dbl[])
      }
      frame True {
      }
    }
  }
  n22 = Array Size(array=w4) -> (size(s)=w10:i32)
  n23 = Decrement(x=w10) -> (x-1=w9:i32)
  n24 = Multiply(x=w4, y=1000.0) -> (x*y=w6:dbl[])
  n25 = Array Max & Min(array=w4) -> (max value=w2:dbl, min value=w3:dbl)  [unwired: 2 out]
  n26 = for {
    N: w9 -> [_]
    tunnel: w6 -> [w54]
    tunnel: [w49] -> w8 mode=indexing
    i -> [w52]
    n27 = Increment(x=w52) -> (x+1=w53:i32)
    n28 = Index Array(array=w54, index=w53) -> (element=w51:dbl)
    n29 = Index Array(array=w54, index=w52) -> (element=w50:dbl)
    n30 = Subtract(x=w51, y=w50) -> (x-y=w49:dbl)
    "Interval time" <- w49
  }
  n31 = Subtract(x=w2, y=w3) -> (x-y=→"전체 시간(s)":dbl)
  n32 = call-poly <vilib>:"Mean.vi"("X"=w8) -> ("mean"=→"평균 Interval time(ms)":dbl)  [unwired: 1 out]
